vi "9401PWM+with+Midi.vi"() -> ()   [LabVIEW 2013]
uses:
  <vilib>/NIOSC/Argument to Float32 Data.vi
  <vilib>/NIOSC/Generate Error.vi
  <vilib>/FPGAPlugInAG/cRIO-9068/niLvFpga_Open_cRIO-9068.vi
  <vilib>/Utility/error.llb/Error Cluster From Error Code.vi
  <vilib>/rvi/errors/niLvFpgaAdjustHostInterfaceError.vi
  <vilib>/FPGAPlugInAG/cRIO-9068/niLvFpga_Close_cRIO-9068.vi
  <vilib>/rvi/interface/nirviOpenFPGA/nirviOpenFPGA.xnode
  FPGA Bitfiles/testscanmode_FPGATarget_FPGA-PWMExample_nwIUPoe6BIw.lvbitx
  FPGA - PWM Example.vi
  <vilib>/rvi/interface/nirviReadWriteControl/nirviReadWriteControl.xnode
  <vilib>/rvi/interface/nirviCloseFPGA/nirviCloseFPGA.xnode
  <vilib>/NIOSC/NI_OSC.lvlib
  NiFpgaLv.dll
  <vilib>/httpClient/LabVIEWHTTPClient.lvlib
panel:
  in  "Descending (F)":bool
  in  "Priority Columns (0)":i32[](array[numeric])=[1, 2]
  out "error midi parse":errorcluster
  out "duration (min:sec)":string="0:00"
  out "Text":string
  out "Track number: name [channel(s) used]":string="Please select a MIDI file..."
  in  "MIDI file (.mid)":path=path "/home/lvuser/bumble_organ.mid"
  out "error urlfile":errorcluster
  in  "url save file":path=path "/home/lvuser/snoop_dogg-the_shiznit.mid"
  in  "shift":i32(slide)=47 scale=-1.0..107.0
  in  "Array":bool[](array[boolean])
  out "/D59":dbl(slide)=0.5
  out "/D60":dbl(slide)=0.5
  out "/D61":dbl(slide)=0.5
  out "/D62":dbl(slide)=0.5
  out "/D63":dbl(slide)=0.5
  in  "OscBool":bool=TRUE
  in  "MidiBool":bool
  out "/D64":dbl(slide)=0.5
  out "error fpga":errorcluster
  out "/D58":dbl
  out "/D57":dbl
  out "/D56":dbl
  out "/D55":dbl
  out "/D54":dbl
  out "/D53":dbl
  out "/D52":dbl
  out "/D51":dbl
  out "/D50":dbl
  out "/D49":dbl
  out "/D48":dbl
  out "/D47":dbl
  out "/D46":dbl
  out "/D45":dbl
  out "/D44":dbl
  out "/D43":dbl
  out "/D42":dbl
  out "/D41":dbl
  out "/D24":dbl
  out "/D23":dbl
  out "/D22":dbl
  out "/D21":dbl
  out "/D20":dbl
  out "/D19":dbl
  out "/D18":dbl
  out "/D17":dbl
  out "/D16":dbl
  out "/D15":dbl
  out "/D14":dbl
  out "/D13":dbl
  out "/D12":dbl
  out "/D11":dbl
  out "/D10":dbl
  out "/D9":dbl
  out "/D8":dbl
  out "/D7":dbl
  out "/D6":dbl
  out "/D5":dbl
  out "/D4":dbl
  out "/D3":dbl
  out "/D2":dbl
  out "/D40":dbl
  out "/D39":dbl
  out "/D38":dbl
  out "/D37":dbl
  out "/D36":dbl
  out "/D35":dbl
  out "/D34":dbl
  out "/D33":dbl
  out "/D1":dbl
  out "/D32":dbl
  out "/D31":dbl
  out "/D30":dbl
  out "/D29":dbl
  out "/D28":dbl
  out "/D27":dbl
  out "/D25":dbl
  out "/D26":dbl
  out "x .and. y?":bool
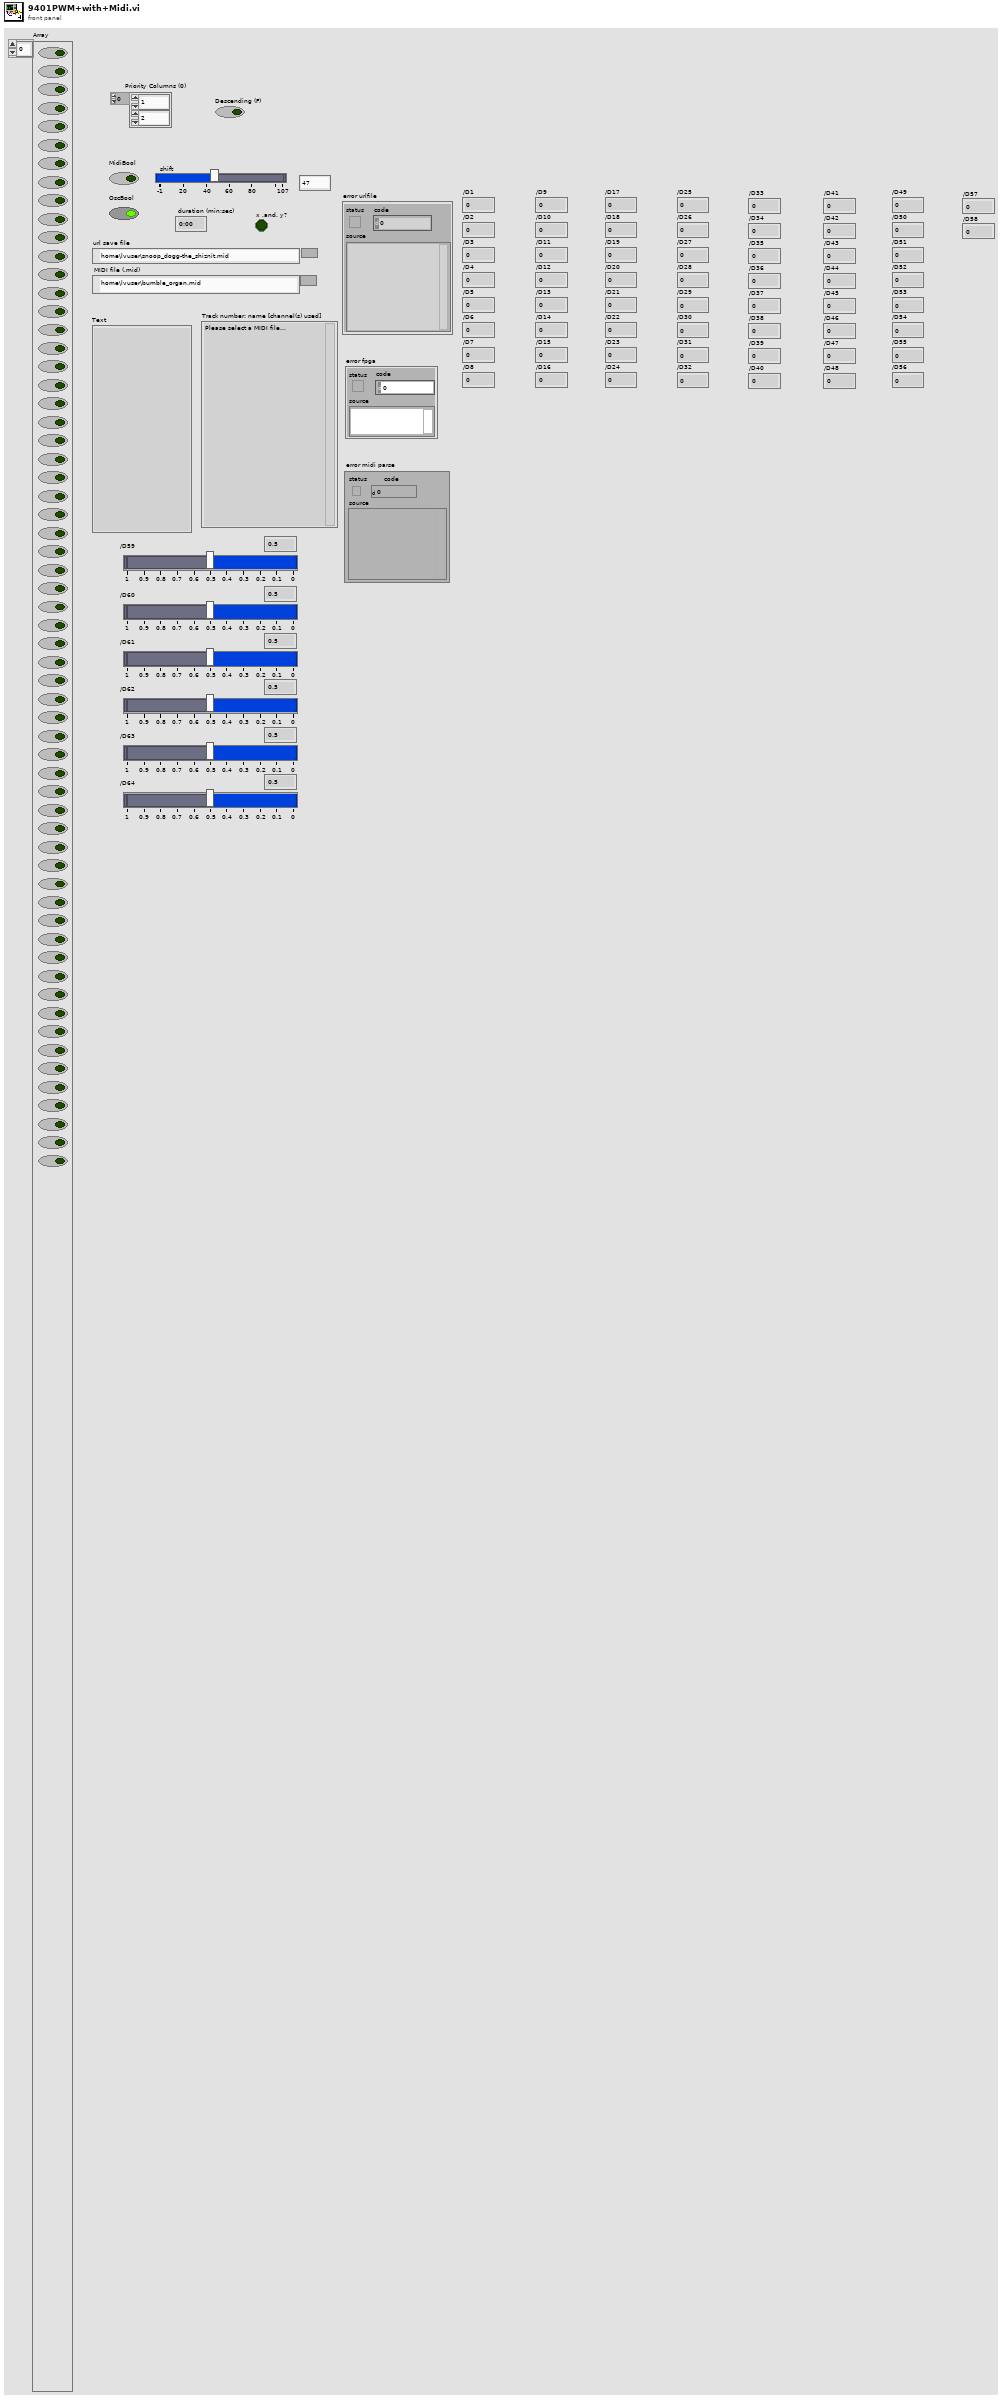
[diagram p1: front panel]
types:
  T1 = typedef "NI_OSC.lvlib/Address Space Node.ctl" = cluster{"parent index":i32, "child indexes":i32[], "address part":string, "method":bool, "data":variant}
  T2 = cluster{"type":u16, "tracks":u16, "ticks per qnote":u16}
  T3 = cluster{"note events":dbl[][], "duration [seconds]":dbl, "track info":string, "text meta-events":string}
  T4 = typedef "NI_OSC.lvlib/Method Dispatching Info.ctl" = cluster{"method address":string, "message":string, "message timetag":u64, "data":variant}
  T5 = typedef "NI_OSC.lvlib/Argument.ctl" = cluster{"argument":string, "type tag":string}
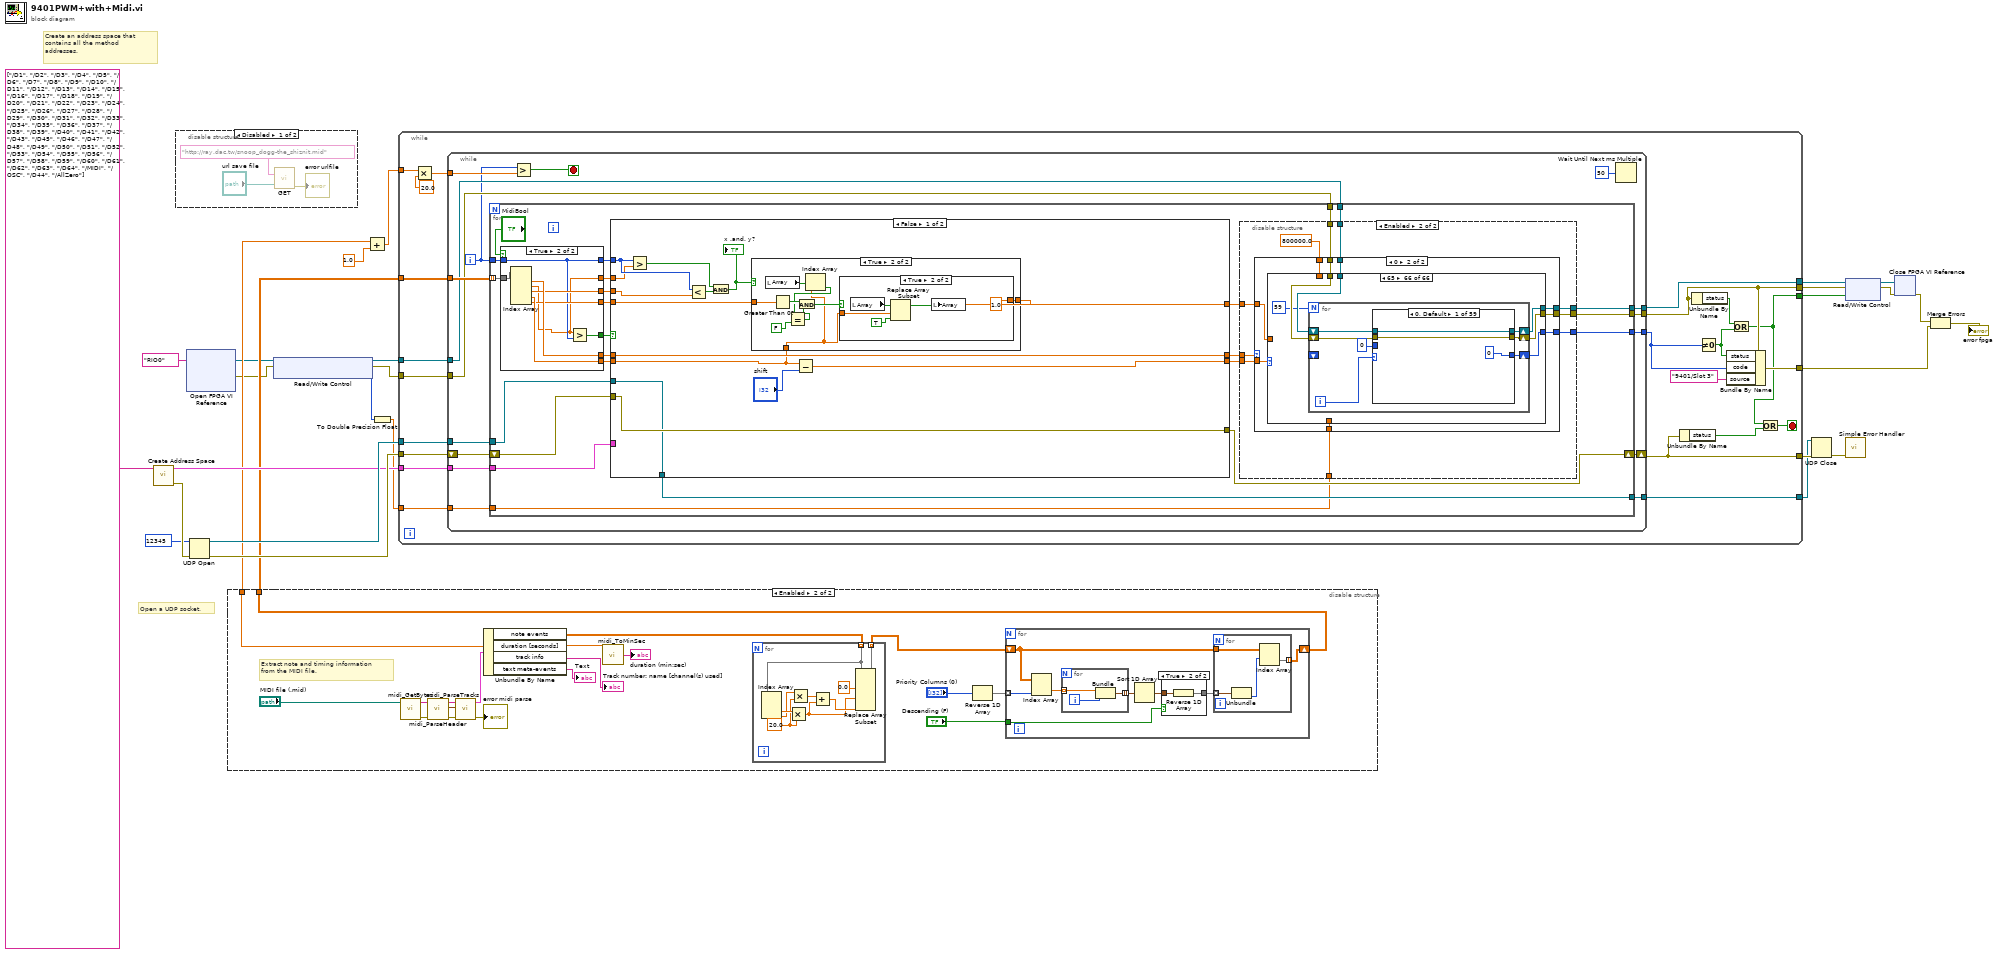
[diagram p0: block diagram]
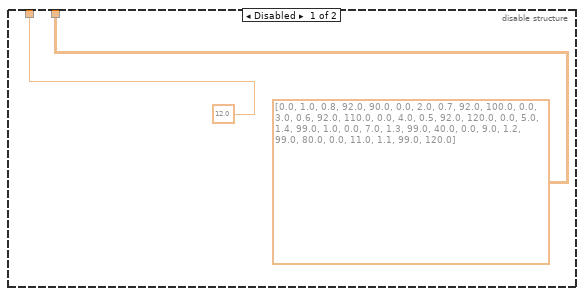
[diagram p3: hidden frame]
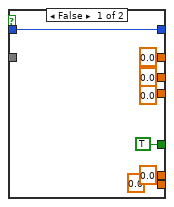
[diagram p5: hidden frame]
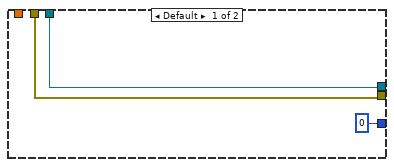
[diagram p7: hidden frame]
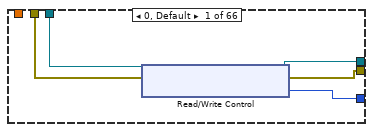
[diagram p8: hidden frame]
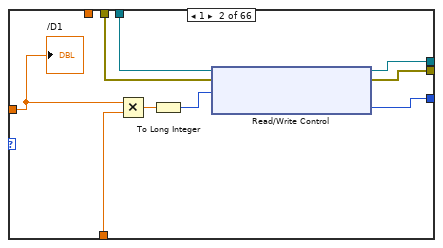
[diagram p9: hidden frame]
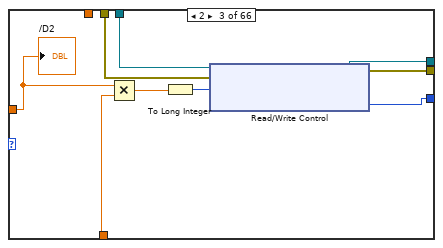
[diagram p10: hidden frame]
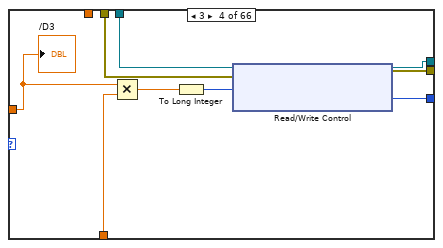
[diagram p11: hidden frame]
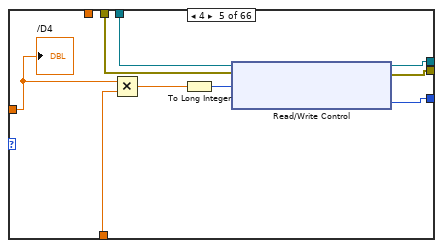
[diagram p12: hidden frame]
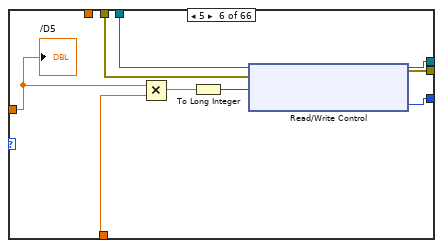
[diagram p13: hidden frame]
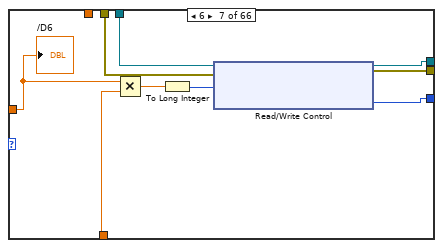
[diagram p14: hidden frame]
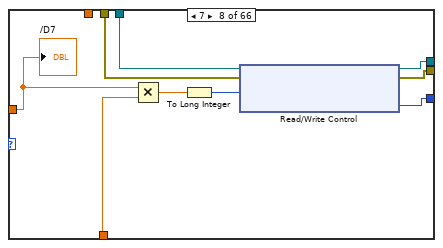
[diagram p15: hidden frame]
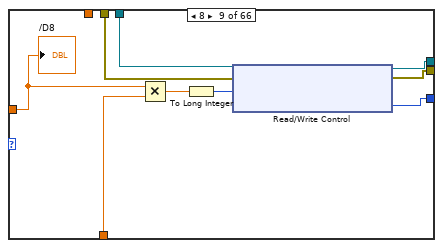
[diagram p16: hidden frame]
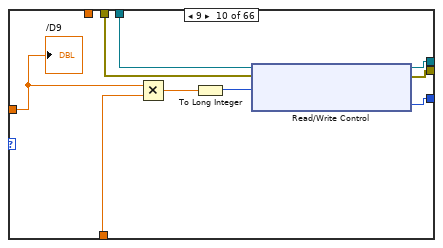
[diagram p17: hidden frame]
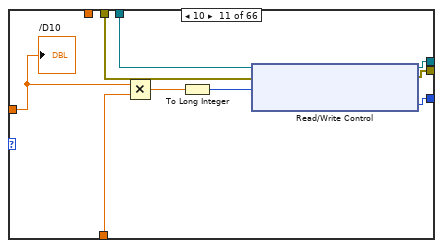
[diagram p18: hidden frame]
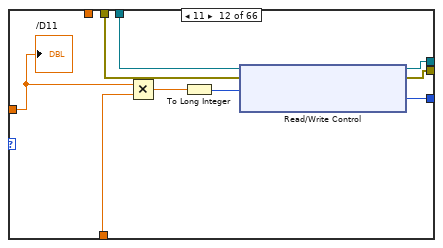
[diagram p19: hidden frame]
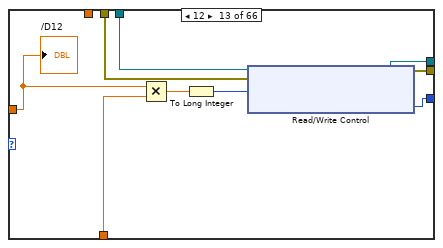
[diagram p20: hidden frame]
diagram:
  # "Open a UDP socket."
  # "Create an address space that contains all the method addresses."
  n1 = call <vilib>:"Create Address Space.vi"("method addresses"=string[] ["/D1", "/D2", "/D3", "/D4", "/D5", "/D6", "/D7", "/D8", "/D9", "/D10", "/D11", "/D12", "/D13", "/D14", "/D15", "/D16", "/D17", "/D18", "/D19", "/D20", "/D21", "/D22", "/D23", "/D24", "/D25", "/D26", "/D27", "/D28", "/D29", "/D30", "/D31", "/D32", "/D33", "/D34", "/D35", "/D36", "/D37", "/D38", "/D39", "/D40", "/D41", "/D42", "/D43", "/D45", "/D46", "/D47", "/D48", "/D49", "/D50", "/D51", "/D52", "/D53", "/D54", "/D55", "/D56", "/D57", "/D58", "/D59", "/D60", "/D61", "/D62", "/D63", "/D64", "/MIDI", "/OSC", "/D44", "/AllZero"]) -> ("error out"=w25:errorcluster, "address space out"=w21:T1[])  [unwired: 9 in]
  n2 = disable-structure shown="Disabled" {
    frame Disabled {
      n3 = call <vilib>:"GET.vi"("output file"="url save file", "url"="http://ray.dac.tw/snoop_dogg-the_shiznit.mid") -> ("error out"=→"error urlfile":errorcluster)  [unwired: 10 in, 3 out]
    }
    frame Enabled {
    }
  }
  n4 = xnode "Open FPGA VI Reference"("resource name"=tag "RIO0") -> ("FPGA VI Reference Out"=w4:refnum<k20>, "error out"=w3:errorcluster)  [unwired: 1 in]
  n5 = UDP Open(8:w25, 11:u16 12345 ("port")) -> (port=w23:refnum<k16>, 0:w22:errorcluster)  [unwired: 3 in, 1 out]
  n6 = disable-structure shown="Enabled" {
    disable-tunnel: [12.0 ("duration [seconds]") w39] -> w20
    disable-tunnel: [dbl[][] [[0.0, 1.0, 0.8, 92.0, 90.0], [0.0, 2.0, 0.7, 92.0, 100.0], [0.0, 3.0, 0.6, 92.0, 110.0], [0.0, 4.0, 0.5, 92.0, 120.0], [0.0, 5.0, 1.4, 99.0, 1.0], [0.0, 7.0, 1.3, 99.0, 40.0], [0.0, 9.0, 1.2, 99.0, 80.0], [0.0, 11.0, 1.1, 99.0, 120.0]] ("note events") w34] -> w19
    frame Disabled {
    }
    frame Enabled {
      # "Extract note and timing information\nfrom the MIDI file."
      n7 = call "midi_GetBytes.vi"("folder name"="MIDI file (.mid)") -> ("error out"=w42:errorcluster, "string"=w49:string)  [unwired: 8 in, 1 out]
      n8 = call "midi_ParseHeader.vi"("error in (no error)"=w42, "string in"=w49) -> ("error out"=w47:errorcluster, "header info"=w43:T2, "string out"=w48:string)  [unwired: 7 in]
      n9 = call "midi_ParseTracks.vi"("error in (no error)"=w47, "header info"=w43, "string in"=w48) -> ("error out"=→"error midi parse":errorcluster, "file contents"=w46:T3)  [unwired: 7 in]
      n10 = Unbundle By Name(w46) -> ("note events"=w40:dbl[][], "duration [seconds]"=w39:dbl, "track info"=→"Track number: name [channel(s) used]":string, "text meta-events"=→"Text":string)
      n11 = call "midi_ToMinSec.vi"("seconds"=w39) -> ("min:sec"=→"duration (min:sec)":string)
      n12 = for {
        tunnel: w40 -> [w76] mode=indexing
        tunnel: [w78] -> w35 mode=indexing
        w74 = 20.0 ("y")
        n13 = Index Array(array=w76) -> (element #2=w75:dbl, element #3=w73:dbl)  [unwired: 3 in, 1 out]
        n14 = Multiply(x=w75, y=w74) -> (x*y=w70:dbl)
        n15 = Multiply(x=w73, y=w74) -> (x*y=w72:dbl)
        n16 = Add(x=w72, y=w70) -> (x+y=w71:dbl)
        n17 = Replace Array Subset(array=w76, new element #1=0.0 ("new element/subarray"), new element #2=w70, new element #3=w71) -> (w78:dbl[])  [unwired: 3 in]
      }
      n18 = Reverse 1D Array(array="Priority Columns (0)") -> (reversed array=w37:i32[])
      n19 = for {
        shift-right: [w53] -> w34
        shift-left: w35 -> [w55]
        tunnel: w37 -> [w52] mode=indexing
        tunnel: "Descending (F)" -> [w54]
        n20 = Index Array(array=w55, index (col)=w52) -> (element=w57:dbl[])  [unwired: 1 in]
        n21 = for {
          tunnel: w57 -> [w67] mode=indexing
          tunnel: [w69] -> w56 mode=indexing
          i -> [w68]
          n22 = Bundle("Numeric"=w67, w68) -> (w69:cluster{"Numeric":dbl, i32})  [unwired: 1 out]
        }
        n23 = Sort 1D Array(array=w56) -> (sorted array=w59:cluster{"Numeric":dbl, i32}[])
        n24 = case shown="True" w54 {
          tunnel: [w60 w61] -> w58
          tunnel: w59 -> [w60 w62]
          frame False {
          }
          frame True {
            n25 = Reverse 1D Array(array=w62) -> (reversed array=w61:cluster{"Numeric":dbl, i32}[])
          }
        }
        n26 = for {
          tunnel: w58 -> [w66] mode=indexing
          tunnel: w55 -> [w65]
          tunnel: [w63] -> w53 mode=indexing
          n27 = Unbundle(w66) -> (w64:i32)  [unwired: 1 out]
          n28 = Index Array(array=w65, index (row)=w64) -> (element=w63:dbl[])  [unwired: 1 in]
        }
      }
    }
  }
  n29 = xnode "Read/Write Control"("FPGA VI Reference In"=w4, "error in"=w3) -> ("FPGA VI Reference Out"=w6:refnum<k20>, "error out"=w5:errorcluster, "PWM Period (Ticks) 0..1"=w2:u32)
  n30 = Add(x=w20, y=1.0) -> (x+y=w28:dbl)
  n31 = To Double Precision Float(number=w2) -> (double precision float=w1:dbl)
  n32 = while {
    tunnel: w19 -> [w100]
    tunnel: w28 -> [w97]
    tunnel: w23 -> [w96]
    tunnel: w22 -> [w95]
    tunnel: w21 -> [w94]
    tunnel: [w80] -> w18
    tunnel: [w93] -> w16
    tunnel: [w89] -> w11
    tunnel: [w88] -> w10
    tunnel: [w82] -> w9
    tunnel: [w86] -> w8
    tunnel: w6 -> [w85]
    tunnel: w5 -> [w84]
    tunnel: w1 -> [w79]
    stop <- w83 stop-if-true
    n33 = Multiply(x=w97, y=20.0) -> (x*y=w98:dbl)
    n34 = while {
      tunnel: w100 -> [w116]
      tunnel: w98 -> [w113]
      tunnel: w94 -> [w110]
      tunnel: w96 -> [w112]
      shift-right: [w109] -> w80
      shift-left: w95 -> [w111]
      tunnel: [w108] -> w93
      tunnel: [w107] -> w88
      tunnel: [w106] -> w89
      tunnel: [w105] -> w87
      tunnel: w85 -> [w104]
      tunnel: w84 -> [w103]
      tunnel: w79 -> [w102]
      i -> [w101]
      stop <- w114 stop-if-true
      n35 = for {
        tunnel: w116 -> [w123] mode=indexing
        tunnel: w101 -> [w125]
        tunnel: w110 -> [w135]
        tunnel: w112 -> [w137]
        shift-right: [w134] -> w109
        shift-left: w111 -> [w136]
        tunnel: [w133] -> w108
        tunnel: [w132] -> w107
        tunnel: [w131] -> w106
        tunnel: [w130] -> w105
        tunnel: w104 -> [w129]
        tunnel: w103 -> [w128]
        tunnel: w102 -> [w127]
        n36 = case shown="True" "MidiBool" {
          tunnel: w125 -> [w147 w149]
          tunnel: [w147 w149] -> w124
          tunnel: w123 -> [_ w155]
          tunnel: [0.0 ("Numeric") w154] -> w122
          tunnel: [0.0 ("Numeric") w153] -> w121
          tunnel: [0.0 w148] -> w120
          tunnel: [0.0 ("Numeric") w152] -> w119
          tunnel: [0.0 ("Numeric") w151] -> w118
          tunnel: [TRUE w150] -> w117
          frame False {
          }
          frame True {
            n37 = Index Array(array=w155) -> (element #1=w153:dbl, element #2=w148:dbl, element #3=w152:dbl, element #4=w154:dbl, element #5=w151:dbl)  [unwired: 5 in]
            n38 = Greater?(x=w148, y=w149) -> (0:w150:bool)
          }
        }
        n39 = case shown="False" w117 {
          tunnel: w118 -> [w1221 _]
          tunnel: w124 -> [w1226 _]
          tunnel: w120 -> [w1225 _]
          tunnel: w119 -> [w1216 _]
          tunnel: w122 -> [w1215 _]
          tunnel: w121 -> [w1218 _]
          tunnel: [w1218 0.0 ("Numeric")] -> w140
          tunnel: [w1217 w1263] -> w139
          tunnel: [w1219 w1259] -> w138
          tunnel: w137 -> [w1223 w1265]
          tunnel: w136 -> [w1224 w1264]
          tunnel: w135 -> [_ w1258]
          tunnel: [w1224 w1262] -> w134
          tunnel: [w1223 w1261] -> w133
          frame False {
            n40 = Greater?(x=w1226, y=w1225) -> (0:w1228:bool)
            n41 = Less?(x=w1226, y=w1216) -> (x < y?=w1227:bool)
            n42 = And(x=w1228, y=w1227) -> (x .and. y?=w1220:bool)
            "x .and. y?" <- w1220
            n43 = case shown="True" w1220 {
              tunnel: w1221 -> [_ w1244]
              tunnel: [w1232 w1241] -> w1219
              tunnel: w1215 -> [w1229 w1240]
              frame False {
                n44 = Index Array(array="Array", index=w1229) -> (element=w1234:bool)
                n45 = Equal?(x=w1234, y=TRUE) -> (x = y?=w1231:bool)
                n46 = case shown="True" w1231 {
                  tunnel: [_ 0.0] -> w1232
                  tunnel: w1229 -> [_ w1238]
                  tunnel: "Array" -> [_ w1237]
                  frame False {
                  }
                  frame True {
                    n47 = Replace Array Subset(array=w1237, new element=FALSE ("new element/subarray"), index=w1238) -> (w1235:bool[])
                    n48 = local write "Array"(w1235) -> ()
                  }
                }
              }
              frame True {
                n49 = local read "Array"() -> (w1248:bool[])
                n50 = Greater Than 0?(x=w1244) -> (x > 0?=w1246:bool)
                n51 = Index Array(array=w1248, index=w1240) -> (element=w1243:bool)
                n52 = Equal?(x=w1243, y=FALSE ("x")) -> (x = y?=w1245:bool)
                n53 = And(x=w1246, y=w1245) -> (x .and. y?=w1247:bool)
                n54 = case shown="True" w1247 {
                  tunnel: [_ 1.0] -> w1241
                  tunnel: w1240 -> [_ w1249]
                  frame False {
                  }
                  frame True {
                    n55 = local read "Array"() -> (w1251:bool[])
                    n56 = Replace Array Subset(array=w1251, new element=TRUE ("new element/subarray"), index=w1249) -> (w1250:bool[])
                    n57 = local write "Array"(w1250) -> ()
                  }
                }
              }
            }
            n58 = Subtract(x=w1215, y="shift") -> (x-y=w1217:dbl)
          }
          frame True {
            n59 = UDP Read(connection ID=w1265, timeout ms (25000)=0, 8:w1264) -> (data out=w1257:string, error out=w1256:errorcluster, 3:w1261:refnum<k16>)  [unwired: 1 in, 2 out]
            n60 = call <vilib>:"Dispatch All Messages.vi"("error in"=w1256, "packet"=w1257, "address space in"=w1258) -> ("error out"=w1255:errorcluster, "method dispatching info"=w1254:T4[])  [unwired: 6 in, 1 out]
            n61 = case shown="No Error" w1255 {
              selector: w1255 -> [w1268 w2007]
              tunnel: [w1272 w2006] -> w1262
              tunnel: [w1271 0] -> w1260
              tunnel: [w1270 0] -> w1263
              tunnel: w1254 -> [w1269 _]
              frame No Error {
                # "Find all method addresses that match the incoming message(s)."
                n62 = for {
                  tunnel: w1269 -> [w1279] mode=indexing
                  shift-right: [w1277] -> w1272
                  shift-left: w1268 -> [w1278]
                  tunnel: [w1274] -> w1271
                  tunnel: [w1273] -> w1270
                  n63 = Unbundle By Name(w1279) -> ("method address"=w1276:string, "message"=w1275:string)
                  n64 = case shown="\"/AllZero\"" w1276 {
                    tunnel: w1278 -> [w1282 w1291 w1302 w1313 w1324 w1335 w1346 w1357 w1368 w1374 w1385 w1397 w1409 w1419 w1430 w1440 w1452 w1464 w1474 w1485 w1496 w1507 w1518 w1529 w1540 w1551 w1562 w1573 w1584 w1595 w1606 w1617 w1628 w1639 w1650 w1661 w1672 w1683 w1694 w1705 w1716 w1727 w1738 w1749 w1760 w1771 w1782 w1793 w1804 w1815 w1825 w1836 w1848 w1858 w1869 w1881 w1891 w1902 w1913 w1923 w1931 w1939 w1947 w1955 w1964 w1974 w1986 w1998]
                    tunnel: [w1282 w1287 w1298 w1309 w1320 w1331 w1342 w1353 w1363 w1376 w1387 w1396 w1408 w1418 w1429 w1442 w1451 w1462 w1473 w1484 w1495 w1506 w1517 w1528 w1539 w1550 w1561 w1572 w1583 w1594 w1605 w1616 w1627 w1638 w1649 w1660 w1671 w1682 w1693 w1704 w1715 w1726 w1737 w1748 w1759 w1770 w1781 w1792 w1803 w1814 w1827 w1838 w1849 w1860 w1871 w1882 w1893 w1904 w1915 w1925 w1933 w1941 w1949 w1957 w1965 w1973 w1985 w1997] -> w1277
                    tunnel: w1275 -> [_ w1286 w1297 w1308 w1319 w1330 w1341 w1352 w1365 w1375 w1386 w1398 w1407 w1420 w1431 w1441 w1453 w1463 w1475 w1486 w1497 w1508 w1519 w1530 w1541 w1552 w1563 w1574 w1585 w1596 w1607 w1618 w1629 w1640 w1651 w1662 w1673 w1684 w1695 w1706 w1717 w1728 w1739 w1750 w1761 w1772 w1783 w1794 w1805 w1816 w1826 w1837 w1847 w1859 w1870 w1880 w1892 w1903 w1914 w1924 w1932 w1940 w1948 w1956 w1963 w1975 w1987 w1996]
                    tunnel: [0 ("int32 data") w1283 w1294 w1305 w1316 w1327 w1338 w1349 w1360 w1371 w1382 w1393 w1404 w1415 w1426 w1437 w1448 w1459 w1470 w1481 w1492 w1503 w1514 w1525 w1536 w1547 w1558 w1569 w1580 w1591 w1602 w1613 w1624 w1635 w1646 w1657 w1668 w1679 w1690 w1701 w1712 w1723 w1734 w1745 w1756 w1767 w1778 w1789 w1800 w1811 w1822 w1833 w1844 w1855 w1866 w1877 w1888 w1899 w1910 w1921 w1929 w1938 w1946 w1954 w1961 0 ("int32 data") 0 ("int32 data") w1994] -> w1274
                    tunnel: [0 w1285 w1296 w1307 w1318 w1328 w1340 w1351 w1362 w1373 w1384 w1395 w1406 w1417 w1428 w1439 w1449 w1461 w1472 w1483 w1494 w1505 w1516 w1527 w1538 w1549 w1560 w1571 w1582 w1593 w1604 w1615 w1626 w1637 w1648 w1659 w1670 w1681 w1692 w1703 w1714 w1725 w1736 w1747 w1758 w1769 w1780 w1791 w1802 w1813 w1824 w1835 w1846 w1857 w1868 w1878 w1889 w1900 w1911 59 60 61 62 63 64 0 0 w1995] -> w1273
                    frame Default {
                    }
                    frame "/D1" {
                      n65 = call <vilib>:"Parse Message.vi"("error in"=w1291, "message"=w1286) -> ("error out"=w1288:errorcluster, "arguments"=w1290:T5[])  [unwired: 7 in, 1 out]
                      n66 = Index Array(array=w1290) -> (element=w1289:T5)  [unwired: 1 in]
                      n67 = call-poly <vilib>:"Argument to Data.vi"("error in"=w1288, "float32 argument"=w1289) -> ("error out"=w1287:errorcluster, "float32 data"=w1283:sgl)  [unwired: 8 in]
                      n68 = local read "OscBool"() -> (w1284:bool)
                      n69 = case shown="True" w1284 {
                        tunnel: [0 1] -> w1285
                        frame False {
                        }
                        frame True {
                        }
                      }
                    }
                    frame "/D2" {
                      n70 = call <vilib>:"Parse Message.vi"("error in"=w1302, "message"=w1297) -> ("error out"=w1299:errorcluster, "arguments"=w1301:T5[])  [unwired: 7 in, 1 out]
                      n71 = Index Array(array=w1301) -> (element=w1300:T5)  [unwired: 1 in]
                      n72 = call-poly <vilib>:"Argument to Data.vi"("error in"=w1299, "float32 argument"=w1300) -> ("error out"=w1298:errorcluster, "float32 data"=w1294:sgl)  [unwired: 8 in]
                      n73 = local read "OscBool"() -> (w1295:bool)
                      n74 = case shown="True" w1295 {
                        tunnel: [0 2] -> w1296
                        frame False {
                        }
                        frame True {
                        }
                      }
                    }
                    frame "/D3" {
                      n75 = local read "OscBool"() -> (w1306:bool)
                      n76 = call <vilib>:"Parse Message.vi"("error in"=w1313, "message"=w1308) -> ("error out"=w1310:errorcluster, "arguments"=w1312:T5[])  [unwired: 7 in, 1 out]
                      n77 = Index Array(array=w1312) -> (element=w1311:T5)  [unwired: 1 in]
                      n78 = case shown="False" w1306 {
                        tunnel: [0 3] -> w1307
                        frame False {
                        }
                        frame True {
                        }
                      }
                      n79 = call-poly <vilib>:"Argument to Data.vi"("error in"=w1310, "float32 argument"=w1311) -> ("error out"=w1309:errorcluster, "float32 data"=w1305:sgl)  [unwired: 8 in]
                    }
                    frame "/D4" {
                      n80 = local read "OscBool"() -> (w1317:bool)
                      n81 = call <vilib>:"Parse Message.vi"("error in"=w1324, "message"=w1319) -> ("error out"=w1321:errorcluster, "arguments"=w1323:T5[])  [unwired: 7 in, 1 out]
                      n82 = Index Array(array=w1323) -> (element=w1322:T5)  [unwired: 1 in]
                      n83 = case shown="True" w1317 {
                        tunnel: [0 4] -> w1318
                        frame False {
                        }
                        frame True {
                        }
                      }
                      n84 = call-poly <vilib>:"Argument to Data.vi"("error in"=w1321, "float32 argument"=w1322) -> ("error out"=w1320:errorcluster, "float32 data"=w1316:sgl)  [unwired: 8 in]
                    }
                    frame "/D5" {
                      n85 = call <vilib>:"Parse Message.vi"("error in"=w1335, "message"=w1330) -> ("error out"=w1332:errorcluster, "arguments"=w1334:T5[])  [unwired: 7 in, 1 out]
                      n86 = Index Array(array=w1334) -> (element=w1333:T5)  [unwired: 1 in]
                      n87 = call-poly <vilib>:"Argument to Data.vi"("error in"=w1332, "float32 argument"=w1333) -> ("error out"=w1331:errorcluster, "float32 data"=w1327:sgl)  [unwired: 8 in]
                      n88 = local read "OscBool"() -> (w1329:bool)
                      n89 = case shown="True" w1329 {
                        tunnel: [0 5] -> w1328
                        frame False {
                        }
                        frame True {
                        }
                      }
                    }
                    frame "/D6" {
                      n90 = call <vilib>:"Parse Message.vi"("error in"=w1346, "message"=w1341) -> ("error out"=w1343:errorcluster, "arguments"=w1345:T5[])  [unwired: 7 in, 1 out]
                      n91 = Index Array(array=w1345) -> (element=w1344:T5)  [unwired: 1 in]
                      n92 = call-poly <vilib>:"Argument to Data.vi"("error in"=w1343, "float32 argument"=w1344) -> ("error out"=w1342:errorcluster, "float32 data"=w1338:sgl)  [unwired: 8 in]
                      n93 = local read "OscBool"() -> (w1339:bool)
                      n94 = case shown="True" w1339 {
                        tunnel: [0 6] -> w1340
                        frame False {
                        }
                        frame True {
                        }
                      }
                    }
                    frame "/D7" {
                      n95 = local read "OscBool"() -> (w1350:bool)
                      n96 = call <vilib>:"Parse Message.vi"("error in"=w1357, "message"=w1352) -> ("error out"=w1354:errorcluster, "arguments"=w1356:T5[])  [unwired: 7 in, 1 out]
                      n97 = Index Array(array=w1356) -> (element=w1355:T5)  [unwired: 1 in]
                      n98 = case shown="True" w1350 {
                        tunnel: [0 7] -> w1351
                        frame False {
                        }
                        frame True {
                        }
                      }
                      n99 = call-poly <vilib>:"Argument to Data.vi"("error in"=w1354, "float32 argument"=w1355) -> ("error out"=w1353:errorcluster, "float32 data"=w1349:sgl)  [unwired: 8 in]
                    }
                    frame "/D8" {
                      n100 = call <vilib>:"Parse Message.vi"("error in"=w1368, "message"=w1365) -> ("error out"=w1364:errorcluster, "arguments"=w1367:T5[])  [unwired: 7 in, 1 out]
                      n101 = local read "OscBool"() -> (w1361:bool)
                      n102 = Index Array(array=w1367) -> (element=w1366:T5)  [unwired: 1 in]
                      n103 = case shown="True" w1361 {
                        tunnel: [0 8] -> w1362
                        frame False {
                        }
                        frame True {
                        }
                      }
                      n104 = call-poly <vilib>:"Argument to Data.vi"("error in"=w1364, "float32 argument"=w1366) -> ("error out"=w1363:errorcluster, "float32 data"=w1360:sgl)  [unwired: 8 in]
                    }
                    frame "/D9" {
                      n105 = local read "OscBool"() -> (w1372:bool)
                      n106 = call <vilib>:"Parse Message.vi"("error in"=w1374, "message"=w1375) -> ("error out"=w1377:errorcluster, "arguments"=w1379:T5[])  [unwired: 7 in, 1 out]
                      n107 = case shown="True" w1372 {
                        tunnel: [0 9] -> w1373
                        frame False {
                        }
                        frame True {
                        }
                      }
                      n108 = Index Array(array=w1379) -> (element=w1378:T5)  [unwired: 1 in]
                      n109 = call-poly <vilib>:"Argument to Data.vi"("error in"=w1377, "float32 argument"=w1378) -> ("error out"=w1376:errorcluster, "float32 data"=w1371:sgl)  [unwired: 8 in]
                    }
                    frame "/D10" {
                      n110 = local read "OscBool"() -> (w1383:bool)
                      n111 = call <vilib>:"Parse Message.vi"("error in"=w1385, "message"=w1386) -> ("error out"=w1390:errorcluster, "arguments"=w1388:T5[])  [unwired: 7 in, 1 out]
                      n112 = case shown="True" w1383 {
                        tunnel: [0 10] -> w1384
                        frame False {
                        }
                        frame True {
                        }
                      }
                      n113 = Index Array(array=w1388) -> (element=w1389:T5)  [unwired: 1 in]
                      n114 = call-poly <vilib>:"Argument to Data.vi"("error in"=w1390, "float32 argument"=w1389) -> ("error out"=w1387:errorcluster, "float32 data"=w1382:sgl)  [unwired: 8 in]
                    }
                    frame "/D11" {
                      n115 = local read "OscBool"() -> (w1394:bool)
                      n116 = call <vilib>:"Parse Message.vi"("error in"=w1397, "message"=w1398) -> ("error out"=w1399:errorcluster, "arguments"=w1401:T5[])  [unwired: 7 in, 1 out]
                      n117 = case shown="True" w1394 {
                        tunnel: [0 11] -> w1395
                        frame False {
                        }
                        frame True {
                        }
                      }
                      n118 = Index Array(array=w1401) -> (element=w1400:T5)  [unwired: 1 in]
                      n119 = call-poly <vilib>:"Argument to Data.vi"("error in"=w1399, "float32 argument"=w1400) -> ("error out"=w1396:errorcluster, "float32 data"=w1393:sgl)  [unwired: 8 in]
                    }
                    frame "/D12" {
                      n120 = local read "OscBool"() -> (w1405:bool)
                      n121 = call <vilib>:"Parse Message.vi"("error in"=w1409, "message"=w1407) -> ("error out"=w1410:errorcluster, "arguments"=w1412:T5[])  [unwired: 7 in, 1 out]
                      n122 = case shown="True" w1405 {
                        tunnel: [0 12] -> w1406
                        frame False {
                        }
                        frame True {
                        }
                      }
                      n123 = Index Array(array=w1412) -> (element=w1411:T5)  [unwired: 1 in]
                      n124 = call-poly <vilib>:"Argument to Data.vi"("error in"=w1410, "float32 argument"=w1411) -> ("error out"=w1408:errorcluster, "float32 data"=w1404:sgl)  [unwired: 8 in]
                    }
                    frame "/D13" {
                      n125 = local read "OscBool"() -> (w1416:bool)
                      n126 = call <vilib>:"Parse Message.vi"("error in"=w1419, "message"=w1420) -> ("error out"=w1423:errorcluster, "arguments"=w1421:T5[])  [unwired: 7 in, 1 out]
                      n127 = case shown="True" w1416 {
                        tunnel: [0 13] -> w1417
                        frame False {
                        }
                        frame True {
                        }
                      }
                      n128 = Index Array(array=w1421) -> (element=w1422:T5)  [unwired: 1 in]
                      n129 = call-poly <vilib>:"Argument to Data.vi"("error in"=w1423, "float32 argument"=w1422) -> ("error out"=w1418:errorcluster, "float32 data"=w1415:sgl)  [unwired: 8 in]
                    }
                    frame "/D14" {
                      n130 = local read "OscBool"() -> (w1427:bool)
                      n131 = call <vilib>:"Parse Message.vi"("error in"=w1430, "message"=w1431) -> ("error out"=w1434:errorcluster, "arguments"=w1432:T5[])  [unwired: 7 in, 1 out]
                      n132 = case shown="True" w1427 {
                        tunnel: [0 14] -> w1428
                        frame False {
                        }
                        frame True {
                        }
                      }
                      n133 = Index Array(array=w1432) -> (element=w1433:T5)  [unwired: 1 in]
                      n134 = call-poly <vilib>:"Argument to Data.vi"("error in"=w1434, "float32 argument"=w1433) -> ("error out"=w1429:errorcluster, "float32 data"=w1426:sgl)  [unwired: 8 in]
                    }
                    frame "/D15" {
                      n135 = local read "OscBool"() -> (w1438:bool)
                      n136 = call <vilib>:"Parse Message.vi"("error in"=w1440, "message"=w1441) -> ("error out"=w1443:errorcluster, "arguments"=w1445:T5[])  [unwired: 7 in, 1 out]
                      n137 = case shown="True" w1438 {
                        tunnel: [0 15] -> w1439
                        frame False {
                        }
                        frame True {
                        }
                      }
                      n138 = Index Array(array=w1445) -> (element=w1444:T5)  [unwired: 1 in]
                      n139 = call-poly <vilib>:"Argument to Data.vi"("error in"=w1443, "float32 argument"=w1444) -> ("error out"=w1442:errorcluster, "float32 data"=w1437:sgl)  [unwired: 8 in]
                    }
                    frame "/D16" {
                      n140 = local read "OscBool"() -> (w1450:bool)
                      n141 = call <vilib>:"Parse Message.vi"("error in"=w1452, "message"=w1453) -> ("error out"=w1454:errorcluster, "arguments"=w1456:T5[])  [unwired: 7 in, 1 out]
                      n142 = case shown="True" w1450 {
                        tunnel: [0 16] -> w1449
                        frame False {
                        }
                        frame True {
                        }
                      }
                      n143 = Index Array(array=w1456) -> (element=w1455:T5)  [unwired: 1 in]
                      n144 = call-poly <vilib>:"Argument to Data.vi"("error in"=w1454, "float32 argument"=w1455) -> ("error out"=w1451:errorcluster, "float32 data"=w1448:sgl)  [unwired: 8 in]
                    }
                    frame "/D17" {
                      n145 = local read "OscBool"() -> (w1460:bool)
                      n146 = call <vilib>:"Parse Message.vi"("error in"=w1464, "message"=w1463) -> ("error out"=w1465:errorcluster, "arguments"=w1467:T5[])  [unwired: 7 in, 1 out]
                      n147 = case shown="True" w1460 {
                        tunnel: [0 17] -> w1461
                        frame False {
                        }
                        frame True {
                        }
                      }
                      n148 = Index Array(array=w1467) -> (element=w1466:T5)  [unwired: 1 in]
                      n149 = call-poly <vilib>:"Argument to Data.vi"("error in"=w1465, "float32 argument"=w1466) -> ("error out"=w1462:errorcluster, "float32 data"=w1459:sgl)  [unwired: 8 in]
                    }
                    frame "/D18" {
                      n150 = local read "OscBool"() -> (w1471:bool)
                      n151 = call <vilib>:"Parse Message.vi"("error in"=w1474, "message"=w1475) -> ("error out"=w1476:errorcluster, "arguments"=w1478:T5[])  [unwired: 7 in, 1 out]
                      n152 = case shown="True" w1471 {
                        tunnel: [0 18] -> w1472
                        frame False {
                        }
                        frame True {
                        }
                      }
                      n153 = Index Array(array=w1478) -> (element=w1477:T5)  [unwired: 1 in]
                      n154 = call-poly <vilib>:"Argument to Data.vi"("error in"=w1476, "float32 argument"=w1477) -> ("error out"=w1473:errorcluster, "float32 data"=w1470:sgl)  [unwired: 8 in]
                    }
                    frame "/D19" {
                      n155 = local read "OscBool"() -> (w1482:bool)
                      n156 = call <vilib>:"Parse Message.vi"("error in"=w1485, "message"=w1486) -> ("error out"=w1487:errorcluster, "arguments"=w1489:T5[])  [unwired: 7 in, 1 out]
                      n157 = case shown="True" w1482 {
                        tunnel: [0 19] -> w1483
                        frame False {
                        }
                        frame True {
                        }
                      }
                      n158 = Index Array(array=w1489) -> (element=w1488:T5)  [unwired: 1 in]
                      n159 = call-poly <vilib>:"Argument to Data.vi"("error in"=w1487, "float32 argument"=w1488) -> ("error out"=w1484:errorcluster, "float32 data"=w1481:sgl)  [unwired: 8 in]
                    }
                    frame "/D20" {
                      n160 = local read "OscBool"() -> (w1493:bool)
                      n161 = call <vilib>:"Parse Message.vi"("error in"=w1496, "message"=w1497) -> ("error out"=w1498:errorcluster, "arguments"=w1500:T5[])  [unwired: 7 in, 1 out]
                      n162 = case shown="False" w1493 {
                        tunnel: [0 20] -> w1494
                        frame False {
                        }
                        frame True {
                        }
                      }
                      n163 = Index Array(array=w1500) -> (element=w1499:T5)  [unwired: 1 in]
                      n164 = call-poly <vilib>:"Argument to Data.vi"("error in"=w1498, "float32 argument"=w1499) -> ("error out"=w1495:errorcluster, "float32 data"=w1492:sgl)  [unwired: 8 in]
                    }
                    frame "/D21" {
                      n165 = local read "OscBool"() -> (w1504:bool)
                      n166 = call <vilib>:"Parse Message.vi"("error in"=w1507, "message"=w1508) -> ("error out"=w1509:errorcluster, "arguments"=w1511:T5[])  [unwired: 7 in, 1 out]
                      n167 = case shown="True" w1504 {
                        tunnel: [0 21] -> w1505
                        frame False {
                        }
                        frame True {
                        }
                      }
                      n168 = Index Array(array=w1511) -> (element=w1510:T5)  [unwired: 1 in]
                      n169 = call-poly <vilib>:"Argument to Data.vi"("error in"=w1509, "float32 argument"=w1510) -> ("error out"=w1506:errorcluster, "float32 data"=w1503:sgl)  [unwired: 8 in]
                    }
                    frame "/D22" {
                      n170 = local read "OscBool"() -> (w1515:bool)
                      n171 = call <vilib>:"Parse Message.vi"("error in"=w1518, "message"=w1519) -> ("error out"=w1520:errorcluster, "arguments"=w1522:T5[])  [unwired: 7 in, 1 out]
                      n172 = case shown="True" w1515 {
                        tunnel: [0 22] -> w1516
                        frame False {
                        }
                        frame True {
                        }
                      }
                      n173 = Index Array(array=w1522) -> (element=w1521:T5)  [unwired: 1 in]
                      n174 = call-poly <vilib>:"Argument to Data.vi"("error in"=w1520, "float32 argument"=w1521) -> ("error out"=w1517:errorcluster, "float32 data"=w1514:sgl)  [unwired: 8 in]
                    }
                    frame "/D23" {
                      n175 = local read "OscBool"() -> (w1526:bool)
                      n176 = call <vilib>:"Parse Message.vi"("error in"=w1529, "message"=w1530) -> ("error out"=w1533:errorcluster, "arguments"=w1531:T5[])  [unwired: 7 in, 1 out]
                      n177 = case shown="True" w1526 {
                        tunnel: [0 23] -> w1527
                        frame False {
                        }
                        frame True {
                        }
                      }
                      n178 = Index Array(array=w1531) -> (element=w1532:T5)  [unwired: 1 in]
                      n179 = call-poly <vilib>:"Argument to Data.vi"("error in"=w1533, "float32 argument"=w1532) -> ("error out"=w1528:errorcluster, "float32 data"=w1525:sgl)  [unwired: 8 in]
                    }
                    frame "/D24" {
                      n180 = local read "OscBool"() -> (w1537:bool)
                      n181 = call <vilib>:"Parse Message.vi"("error in"=w1540, "message"=w1541) -> ("error out"=w1542:errorcluster, "arguments"=w1544:T5[])  [unwired: 7 in, 1 out]
                      n182 = case shown="True" w1537 {
                        tunnel: [0 24] -> w1538
                        frame False {
                        }
                        frame True {
                        }
                      }
                      n183 = Index Array(array=w1544) -> (element=w1543:T5)  [unwired: 1 in]
                      n184 = call-poly <vilib>:"Argument to Data.vi"("error in"=w1542, "float32 argument"=w1543) -> ("error out"=w1539:errorcluster, "float32 data"=w1536:sgl)  [unwired: 8 in]
                    }
                    frame "/D25" {
                      n185 = local read "OscBool"() -> (w1548:bool)
                      n186 = call <vilib>:"Parse Message.vi"("error in"=w1551, "message"=w1552) -> ("error out"=w1555:errorcluster, "arguments"=w1553:T5[])  [unwired: 7 in, 1 out]
                      n187 = case shown="True" w1548 {
                        tunnel: [0 25] -> w1549
                        frame False {
                        }
                        frame True {
                        }
                      }
                      n188 = Index Array(array=w1553) -> (element=w1554:T5)  [unwired: 1 in]
                      n189 = call-poly <vilib>:"Argument to Data.vi"("error in"=w1555, "float32 argument"=w1554) -> ("error out"=w1550:errorcluster, "float32 data"=w1547:sgl)  [unwired: 8 in]
                    }
                    frame "/D26" {
                      n190 = local read "OscBool"() -> (w1559:bool)
                      n191 = call <vilib>:"Parse Message.vi"("error in"=w1562, "message"=w1563) -> ("error out"=w1564:errorcluster, "arguments"=w1566:T5[])  [unwired: 7 in, 1 out]
                      n192 = case shown="True" w1559 {
                        tunnel: [0 26] -> w1560
                        frame False {
                        }
                        frame True {
                        }
                      }
                      n193 = Index Array(array=w1566) -> (element=w1565:T5)  [unwired: 1 in]
                      n194 = call-poly <vilib>:"Argument to Data.vi"("error in"=w1564, "float32 argument"=w1565) -> ("error out"=w1561:errorcluster, "float32 data"=w1558:sgl)  [unwired: 8 in]
                    }
                    frame "/D27" {
                      n195 = local read "OscBool"() -> (w1570:bool)
                      n196 = call <vilib>:"Parse Message.vi"("error in"=w1573, "message"=w1574) -> ("error out"=w1577:errorcluster, "arguments"=w1575:T5[])  [unwired: 7 in, 1 out]
                      n197 = case shown="True" w1570 {
                        tunnel: [0 27] -> w1571
                        frame False {
                        }
                        frame True {
                        }
                      }
                      n198 = Index Array(array=w1575) -> (element=w1576:T5)  [unwired: 1 in]
                      n199 = call-poly <vilib>:"Argument to Data.vi"("error in"=w1577, "float32 argument"=w1576) -> ("error out"=w1572:errorcluster, "float32 data"=w1569:sgl)  [unwired: 8 in]
                    }
                    frame "/D28" {
                      n200 = local read "OscBool"() -> (w1581:bool)
                      n201 = call <vilib>:"Parse Message.vi"("error in"=w1584, "message"=w1585) -> ("error out"=w1588:errorcluster, "arguments"=w1586:T5[])  [unwired: 7 in, 1 out]
                      n202 = case shown="True" w1581 {
                        tunnel: [0 28] -> w1582
                        frame False {
                        }
                        frame True {
                        }
                      }
                      n203 = Index Array(array=w1586) -> (element=w1587:T5)  [unwired: 1 in]
                      n204 = call-poly <vilib>:"Argument to Data.vi"("error in"=w1588, "float32 argument"=w1587) -> ("error out"=w1583:errorcluster, "float32 data"=w1580:sgl)  [unwired: 8 in]
                    }
                    frame "/D29" {
                      n205 = local read "OscBool"() -> (w1592:bool)
                      n206 = call <vilib>:"Parse Message.vi"("error in"=w1595, "message"=w1596) -> ("error out"=w1597:errorcluster, "arguments"=w1599:T5[])  [unwired: 7 in, 1 out]
                      n207 = case shown="True" w1592 {
                        tunnel: [0 29] -> w1593
                        frame False {
                        }
                        frame True {
                        }
                      }
                      n208 = Index Array(array=w1599) -> (element=w1598:T5)  [unwired: 1 in]
                      n209 = call-poly <vilib>:"Argument to Data.vi"("error in"=w1597, "float32 argument"=w1598) -> ("error out"=w1594:errorcluster, "float32 data"=w1591:sgl)  [unwired: 8 in]
                    }
                    frame "/D30" {
                      n210 = local read "OscBool"() -> (w1603:bool)
                      n211 = call <vilib>:"Parse Message.vi"("error in"=w1606, "message"=w1607) -> ("error out"=w1608:errorcluster, "arguments"=w1610:T5[])  [unwired: 7 in, 1 out]
                      n212 = case shown="True" w1603 {
                        tunnel: [0 30] -> w1604
                        frame False {
                        }
                        frame True {
                        }
                      }
                      n213 = Index Array(array=w1610) -> (element=w1609:T5)  [unwired: 1 in]
                      n214 = call-poly <vilib>:"Argument to Data.vi"("error in"=w1608, "float32 argument"=w1609) -> ("error out"=w1605:errorcluster, "float32 data"=w1602:sgl)  [unwired: 8 in]
                    }
                    frame "/D31" {
                      n215 = local read "OscBool"() -> (w1614:bool)
                      n216 = call <vilib>:"Parse Message.vi"("error in"=w1617, "message"=w1618) -> ("error out"=w1619:errorcluster, "arguments"=w1621:T5[])  [unwired: 7 in, 1 out]
                      n217 = case shown="True" w1614 {
                        tunnel: [0 31] -> w1615
                        frame False {
                        }
                        frame True {
                        }
                      }
                      n218 = Index Array(array=w1621) -> (element=w1620:T5)  [unwired: 1 in]
                      n219 = call-poly <vilib>:"Argument to Data.vi"("error in"=w1619, "float32 argument"=w1620) -> ("error out"=w1616:errorcluster, "float32 data"=w1613:sgl)  [unwired: 8 in]
                    }
                    frame "/D32" {
                      n220 = local read "OscBool"() -> (w1625:bool)
                      n221 = call <vilib>:"Parse Message.vi"("error in"=w1628, "message"=w1629) -> ("error out"=w1630:errorcluster, "arguments"=w1632:T5[])  [unwired: 7 in, 1 out]
                      n222 = case shown="True" w1625 {
                        tunnel: [0 32] -> w1626
                        frame False {
                        }
                        frame True {
                        }
                      }
                      n223 = Index Array(array=w1632) -> (element=w1631:T5)  [unwired: 1 in]
                      n224 = call-poly <vilib>:"Argument to Data.vi"("error in"=w1630, "float32 argument"=w1631) -> ("error out"=w1627:errorcluster, "float32 data"=w1624:sgl)  [unwired: 8 in]
                    }
                    frame "/D33" {
                      n225 = local read "OscBool"() -> (w1636:bool)
                      n226 = call <vilib>:"Parse Message.vi"("error in"=w1639, "message"=w1640) -> ("error out"=w1643:errorcluster, "arguments"=w1641:T5[])  [unwired: 7 in, 1 out]
                      n227 = case shown="True" w1636 {
                        tunnel: [0 33] -> w1637
                        frame False {
                        }
                        frame True {
                        }
                      }
                      n228 = Index Array(array=w1641) -> (element=w1642:T5)  [unwired: 1 in]
                      n229 = call-poly <vilib>:"Argument to Data.vi"("error in"=w1643, "float32 argument"=w1642) -> ("error out"=w1638:errorcluster, "float32 data"=w1635:sgl)  [unwired: 8 in]
                    }
                    frame "/D34" {
                      n230 = local read "OscBool"() -> (w1647:bool)
                      n231 = call <vilib>:"Parse Message.vi"("error in"=w1650, "message"=w1651) -> ("error out"=w1654:errorcluster, "arguments"=w1652:T5[])  [unwired: 7 in, 1 out]
                      n232 = case shown="True" w1647 {
                        tunnel: [0 34] -> w1648
                        frame False {
                        }
                        frame True {
                        }
                      }
                      n233 = Index Array(array=w1652) -> (element=w1653:T5)  [unwired: 1 in]
                      n234 = call-poly <vilib>:"Argument to Data.vi"("error in"=w1654, "float32 argument"=w1653) -> ("error out"=w1649:errorcluster, "float32 data"=w1646:sgl)  [unwired: 8 in]
                    }
                    frame "/D35" {
                      n235 = local read "OscBool"() -> (w1658:bool)
                      n236 = call <vilib>:"Parse Message.vi"("error in"=w1661, "message"=w1662) -> ("error out"=w1663:errorcluster, "arguments"=w1665:T5[])  [unwired: 7 in, 1 out]
                      n237 = case shown="True" w1658 {
                        tunnel: [0 35] -> w1659
                        frame False {
                        }
                        frame True {
                        }
                      }
                      n238 = Index Array(array=w1665) -> (element=w1664:T5)  [unwired: 1 in]
                      n239 = call-poly <vilib>:"Argument to Data.vi"("error in"=w1663, "float32 argument"=w1664) -> ("error out"=w1660:errorcluster, "float32 data"=w1657:sgl)  [unwired: 8 in]
                    }
                    frame "/D36" {
                      n240 = local read "OscBool"() -> (w1669:bool)
                      n241 = case shown="True" w1669 {
                        tunnel: [0 36] -> w1670
                        frame False {
                        }
                        frame True {
                        }
                      }
                      n242 = call <vilib>:"Parse Message.vi"("error in"=w1672, "message"=w1673) -> ("error out"=w1676:errorcluster, "arguments"=w1674:T5[])  [unwired: 7 in, 1 out]
                      n243 = Index Array(array=w1674) -> (element=w1675:T5)  [unwired: 1 in]
                      n244 = call-poly <vilib>:"Argument to Data.vi"("error in"=w1676, "float32 argument"=w1675) -> ("error out"=w1671:errorcluster, "float32 data"=w1668:sgl)  [unwired: 8 in]
                    }
                    frame "/D37" {
                      n245 = local read "OscBool"() -> (w1680:bool)
                      n246 = case shown="True" w1680 {
                        tunnel: [0 37] -> w1681
                        frame False {
                        }
                        frame True {
                        }
                      }
                      n247 = call <vilib>:"Parse Message.vi"("error in"=w1683, "message"=w1684) -> ("error out"=w1685:errorcluster, "arguments"=w1687:T5[])  [unwired: 7 in, 1 out]
                      n248 = Index Array(array=w1687) -> (element=w1686:T5)  [unwired: 1 in]
                      n249 = call-poly <vilib>:"Argument to Data.vi"("error in"=w1685, "float32 argument"=w1686) -> ("error out"=w1682:errorcluster, "float32 data"=w1679:sgl)  [unwired: 8 in]
                    }
                    frame "/D38" {
                      n250 = local read "OscBool"() -> (w1691:bool)
                      n251 = call <vilib>:"Parse Message.vi"("error in"=w1694, "message"=w1695) -> ("error out"=w1696:errorcluster, "arguments"=w1698:T5[])  [unwired: 7 in, 1 out]
                      n252 = case shown="True" w1691 {
                        tunnel: [0 38] -> w1692
                        frame False {
                        }
                        frame True {
                        }
                      }
                      n253 = Index Array(array=w1698) -> (element=w1697:T5)  [unwired: 1 in]
                      n254 = call-poly <vilib>:"Argument to Data.vi"("error in"=w1696, "float32 argument"=w1697) -> ("error out"=w1693:errorcluster, "float32 data"=w1690:sgl)  [unwired: 8 in]
                    }
                    frame "/D39" {
                      n255 = local read "OscBool"() -> (w1702:bool)
                      n256 = call <vilib>:"Parse Message.vi"("error in"=w1705, "message"=w1706) -> ("error out"=w1707:errorcluster, "arguments"=w1709:T5[])  [unwired: 7 in, 1 out]
                      n257 = case shown="True" w1702 {
                        tunnel: [0 39] -> w1703
                        frame False {
                        }
                        frame True {
                        }
                      }
                      n258 = Index Array(array=w1709) -> (element=w1708:T5)  [unwired: 1 in]
                      n259 = call-poly <vilib>:"Argument to Data.vi"("error in"=w1707, "float32 argument"=w1708) -> ("error out"=w1704:errorcluster, "float32 data"=w1701:sgl)  [unwired: 8 in]
                    }
                    frame "/D40" {
                      n260 = local read "OscBool"() -> (w1713:bool)
                      n261 = call <vilib>:"Parse Message.vi"("error in"=w1716, "message"=w1717) -> ("error out"=w1718:errorcluster, "arguments"=w1720:T5[])  [unwired: 7 in, 1 out]
                      n262 = case shown="True" w1713 {
                        tunnel: [0 40] -> w1714
                        frame False {
                        }
                        frame True {
                        }
                      }
                      n263 = Index Array(array=w1720) -> (element=w1719:T5)  [unwired: 1 in]
                      n264 = call-poly <vilib>:"Argument to Data.vi"("error in"=w1718, "float32 argument"=w1719) -> ("error out"=w1715:errorcluster, "float32 data"=w1712:sgl)  [unwired: 8 in]
                    }
                    frame "/D41" {
                      n265 = local read "OscBool"() -> (w1724:bool)
                      n266 = case shown="True" w1724 {
                        tunnel: [0 41] -> w1725
                        frame False {
                        }
                        frame True {
                        }
                      }
                      n267 = call <vilib>:"Parse Message.vi"("error in"=w1727, "message"=w1728) -> ("error out"=w1729:errorcluster, "arguments"=w1731:T5[])  [unwired: 7 in, 1 out]
                      n268 = Index Array(array=w1731) -> (element=w1730:T5)  [unwired: 1 in]
                      n269 = call-poly <vilib>:"Argument to Data.vi"("error in"=w1729, "float32 argument"=w1730) -> ("error out"=w1726:errorcluster, "float32 data"=w1723:sgl)  [unwired: 8 in]
                    }
                    frame "/D42" {
                      n270 = local read "OscBool"() -> (w1735:bool)
                      n271 = call <vilib>:"Parse Message.vi"("error in"=w1738, "message"=w1739) -> ("error out"=w1742:errorcluster, "arguments"=w1740:T5[])  [unwired: 7 in, 1 out]
                      n272 = case shown="True" w1735 {
                        tunnel: [0 42] -> w1736
                        frame False {
                        }
                        frame True {
                        }
                      }
                      n273 = Index Array(array=w1740) -> (element=w1741:T5)  [unwired: 1 in]
                      n274 = call-poly <vilib>:"Argument to Data.vi"("error in"=w1742, "float32 argument"=w1741) -> ("error out"=w1737:errorcluster, "float32 data"=w1734:sgl)  [unwired: 8 in]
                    }
                    frame "/D43" {
                      n275 = local read "OscBool"() -> (w1746:bool)
                      n276 = call <vilib>:"Parse Message.vi"("error in"=w1749, "message"=w1750) -> ("error out"=w1753:errorcluster, "arguments"=w1751:T5[])  [unwired: 7 in, 1 out]
                      n277 = case shown="True" w1746 {
                        tunnel: [0 43] -> w1747
                        frame False {
                        }
                        frame True {
                        }
                      }
                      n278 = Index Array(array=w1751) -> (element=w1752:T5)  [unwired: 1 in]
                      n279 = call-poly <vilib>:"Argument to Data.vi"("error in"=w1753, "float32 argument"=w1752) -> ("error out"=w1748:errorcluster, "float32 data"=w1745:sgl)  [unwired: 8 in]
                    }
                    frame "/D44" {
                      n280 = local read "OscBool"() -> (w1757:bool)
                      n281 = call <vilib>:"Parse Message.vi"("error in"=w1760, "message"=w1761) -> ("error out"=w1764:errorcluster, "arguments"=w1762:T5[])  [unwired: 7 in, 1 out]
                      n282 = case shown="True" w1757 {
                        tunnel: [0 44] -> w1758
                        frame False {
                        }
                        frame True {
                        }
                      }
                      n283 = Index Array(array=w1762) -> (element=w1763:T5)  [unwired: 1 in]
                      n284 = call-poly <vilib>:"Argument to Data.vi"("error in"=w1764, "float32 argument"=w1763) -> ("error out"=w1759:errorcluster, "float32 data"=w1756:sgl)  [unwired: 8 in]
                    }
                    frame "/D45" {
                      n285 = local read "OscBool"() -> (w1768:bool)
                      n286 = call <vilib>:"Parse Message.vi"("error in"=w1771, "message"=w1772) -> ("error out"=w1773:errorcluster, "arguments"=w1775:T5[])  [unwired: 7 in, 1 out]
                      n287 = case shown="True" w1768 {
                        tunnel: [0 45] -> w1769
                        frame False {
                        }
                        frame True {
                        }
                      }
                      n288 = Index Array(array=w1775) -> (element=w1774:T5)  [unwired: 1 in]
                      n289 = call-poly <vilib>:"Argument to Data.vi"("error in"=w1773, "float32 argument"=w1774) -> ("error out"=w1770:errorcluster, "float32 data"=w1767:sgl)  [unwired: 8 in]
                    }
                    frame "/D46" {
                      n290 = local read "OscBool"() -> (w1779:bool)
                      n291 = call <vilib>:"Parse Message.vi"("error in"=w1782, "message"=w1783) -> ("error out"=w1786:errorcluster, "arguments"=w1784:T5[])  [unwired: 7 in, 1 out]
                      n292 = case shown="True" w1779 {
                        tunnel: [0 46] -> w1780
                        frame False {
                        }
                        frame True {
                        }
                      }
                      n293 = Index Array(array=w1784) -> (element=w1785:T5)  [unwired: 1 in]
                      n294 = call-poly <vilib>:"Argument to Data.vi"("error in"=w1786, "float32 argument"=w1785) -> ("error out"=w1781:errorcluster, "float32 data"=w1778:sgl)  [unwired: 8 in]
                    }
                    frame "/D47" {
                      n295 = local read "OscBool"() -> (w1790:bool)
                      n296 = call <vilib>:"Parse Message.vi"("error in"=w1793, "message"=w1794) -> ("error out"=w1795:errorcluster, "arguments"=w1797:T5[])  [unwired: 7 in, 1 out]
                      n297 = case shown="False" w1790 {
                        tunnel: [0 47] -> w1791
                        frame False {
                        }
                        frame True {
                        }
                      }
                      n298 = Index Array(array=w1797) -> (element=w1796:T5)  [unwired: 1 in]
                      n299 = call-poly <vilib>:"Argument to Data.vi"("error in"=w1795, "float32 argument"=w1796) -> ("error out"=w1792:errorcluster, "float32 data"=w1789:sgl)  [unwired: 8 in]
                    }
                    frame "/D48" {
                      n300 = call <vilib>:"Parse Message.vi"("error in"=w1804, "message"=w1805) -> ("error out"=w1806:errorcluster, "arguments"=w1808:T5[])  [unwired: 7 in, 1 out]
                      n301 = Index Array(array=w1808) -> (element=w1807:T5)  [unwired: 1 in]
                      n302 = call-poly <vilib>:"Argument to Data.vi"("error in"=w1806, "float32 argument"=w1807) -> ("error out"=w1803:errorcluster, "float32 data"=w1800:sgl)  [unwired: 8 in]
                      n303 = case shown="True" "OscBool" {
                        tunnel: [0 48] -> w1802
                        frame False {
                        }
                        frame True {
                        }
                      }
                    }
                    frame "/D49" {
                      n304 = local read "OscBool"() -> (w1812:bool)
                      n305 = case shown="True" w1812 {
                        tunnel: [0 49] -> w1813
                        frame False {
                        }
                        frame True {
                        }
                      }
                      n306 = call <vilib>:"Parse Message.vi"("error in"=w1815, "message"=w1816) -> ("error out"=w1819:errorcluster, "arguments"=w1817:T5[])  [unwired: 7 in, 1 out]
                      n307 = Index Array(array=w1817) -> (element=w1818:T5)  [unwired: 1 in]
                      n308 = call-poly <vilib>:"Argument to Data.vi"("error in"=w1819, "float32 argument"=w1818) -> ("error out"=w1814:errorcluster, "float32 data"=w1811:sgl)  [unwired: 8 in]
                    }
                    frame "/D50" {
                      n309 = local read "OscBool"() -> (w1823:bool)
                      n310 = call <vilib>:"Parse Message.vi"("error in"=w1825, "message"=w1826) -> ("error out"=w1828:errorcluster, "arguments"=w1830:T5[])  [unwired: 7 in, 1 out]
                      n311 = case shown="True" w1823 {
                        tunnel: [0 50] -> w1824
                        frame False {
                        }
                        frame True {
                        }
                      }
                      n312 = Index Array(array=w1830) -> (element=w1829:T5)  [unwired: 1 in]
                      n313 = call-poly <vilib>:"Argument to Data.vi"("error in"=w1828, "float32 argument"=w1829) -> ("error out"=w1827:errorcluster, "float32 data"=w1822:sgl)  [unwired: 8 in]
                    }
                    frame "/D51" {
                      n314 = local read "OscBool"() -> (w1834:bool)
                      n315 = case shown="True" w1834 {
                        tunnel: [0 51] -> w1835
                        frame False {
                        }
                        frame True {
                        }
                      }
                      n316 = call <vilib>:"Parse Message.vi"("error in"=w1836, "message"=w1837) -> ("error out"=w1841:errorcluster, "arguments"=w1839:T5[])  [unwired: 7 in, 1 out]
                      n317 = Index Array(array=w1839) -> (element=w1840:T5)  [unwired: 1 in]
                      n318 = call-poly <vilib>:"Argument to Data.vi"("error in"=w1841, "float32 argument"=w1840) -> ("error out"=w1838:errorcluster, "float32 data"=w1833:sgl)  [unwired: 8 in]
                    }
                    frame "/D52" {
                      n319 = local read "OscBool"() -> (w1845:bool)
                      n320 = call <vilib>:"Parse Message.vi"("error in"=w1848, "message"=w1847) -> ("error out"=w1852:errorcluster, "arguments"=w1850:T5[])  [unwired: 7 in, 1 out]
                      n321 = case shown="True" w1845 {
                        tunnel: [0 52] -> w1846
                        frame False {
                        }
                        frame True {
                        }
                      }
                      n322 = Index Array(array=w1850) -> (element=w1851:T5)  [unwired: 1 in]
                      n323 = call-poly <vilib>:"Argument to Data.vi"("error in"=w1852, "float32 argument"=w1851) -> ("error out"=w1849:errorcluster, "float32 data"=w1844:sgl)  [unwired: 8 in]
                    }
                    frame "/D53" {
                      n324 = local read "OscBool"() -> (w1856:bool)
                      n325 = call <vilib>:"Parse Message.vi"("error in"=w1858, "message"=w1859) -> ("error out"=w1863:errorcluster, "arguments"=w1861:T5[])  [unwired: 7 in, 1 out]
                      n326 = case shown="True" w1856 {
                        tunnel: [0 53] -> w1857
                        frame False {
                        }
                        frame True {
                        }
                      }
                      n327 = Index Array(array=w1861) -> (element=w1862:T5)  [unwired: 1 in]
                      n328 = call-poly <vilib>:"Argument to Data.vi"("error in"=w1863, "float32 argument"=w1862) -> ("error out"=w1860:errorcluster, "float32 data"=w1855:sgl)  [unwired: 8 in]
                    }
                    frame "/D54" {
                      n329 = local read "OscBool"() -> (w1867:bool)
                      n330 = case shown="True" w1867 {
                        tunnel: [0 54] -> w1868
                        frame False {
                        }
                        frame True {
                        }
                      }
                      n331 = call <vilib>:"Parse Message.vi"("error in"=w1869, "message"=w1870) -> ("error out"=w1872:errorcluster, "arguments"=w1874:T5[])  [unwired: 7 in, 1 out]
                      n332 = Index Array(array=w1874) -> (element=w1873:T5)  [unwired: 1 in]
                      n333 = call-poly <vilib>:"Argument to Data.vi"("error in"=w1872, "float32 argument"=w1873) -> ("error out"=w1871:errorcluster, "float32 data"=w1866:sgl)  [unwired: 8 in]
                    }
                    frame "/D55" {
                      n334 = local read "OscBool"() -> (w1879:bool)
                      n335 = case shown="True" w1879 {
                        tunnel: [0 55] -> w1878
                        frame False {
                        }
                        frame True {
                        }
                      }
                      n336 = call <vilib>:"Parse Message.vi"("error in"=w1881, "message"=w1880) -> ("error out"=w1885:errorcluster, "arguments"=w1883:T5[])  [unwired: 7 in, 1 out]
                      n337 = Index Array(array=w1883) -> (element=w1884:T5)  [unwired: 1 in]
                      n338 = call-poly <vilib>:"Argument to Data.vi"("error in"=w1885, "float32 argument"=w1884) -> ("error out"=w1882:errorcluster, "float32 data"=w1877:sgl)  [unwired: 8 in]
                    }
                    frame "/D56" {
                      n339 = local read "OscBool"() -> (w1890:bool)
                      n340 = case shown="True" w1890 {
                        tunnel: [0 56] -> w1889
                        frame False {
                        }
                        frame True {
                        }
                      }
                      n341 = call <vilib>:"Parse Message.vi"("error in"=w1891, "message"=w1892) -> ("error out"=w1894:errorcluster, "arguments"=w1896:T5[])  [unwired: 7 in, 1 out]
                      n342 = Index Array(array=w1896) -> (element=w1895:T5)  [unwired: 1 in]
                      n343 = call-poly <vilib>:"Argument to Data.vi"("error in"=w1894, "float32 argument"=w1895) -> ("error out"=w1893:errorcluster, "float32 data"=w1888:sgl)  [unwired: 8 in]
                    }
                    frame "/D57" {
                      n344 = local read "OscBool"() -> (w1901:bool)
                      n345 = case shown="True" w1901 {
                        tunnel: [0 57] -> w1900
                        frame False {
                        }
                        frame True {
                        }
                      }
                      n346 = call <vilib>:"Parse Message.vi"("error in"=w1902, "message"=w1903) -> ("error out"=w1907:errorcluster, "arguments"=w1905:T5[])  [unwired: 7 in, 1 out]
                      n347 = Index Array(array=w1905) -> (element=w1906:T5)  [unwired: 1 in]
                      n348 = call-poly <vilib>:"Argument to Data.vi"("error in"=w1907, "float32 argument"=w1906) -> ("error out"=w1904:errorcluster, "float32 data"=w1899:sgl)  [unwired: 8 in]
                    }
                    frame "/D58" {
                      n349 = local read "OscBool"() -> (w1912:bool)
                      n350 = case shown="True" w1912 {
                        tunnel: [0 58] -> w1911
                        frame False {
                        }
                        frame True {
                        }
                      }
                      n351 = call <vilib>:"Parse Message.vi"("error in"=w1913, "message"=w1914) -> ("error out"=w1918:errorcluster, "arguments"=w1916:T5[])  [unwired: 7 in, 1 out]
                      n352 = Index Array(array=w1916) -> (element=w1917:T5)  [unwired: 1 in]
                      n353 = call-poly <vilib>:"Argument to Data.vi"("error in"=w1918, "float32 argument"=w1917) -> ("error out"=w1915:errorcluster, "float32 data"=w1910:sgl)  [unwired: 8 in]
                    }
                    frame "/D59" {
                      n354 = call <vilib>:"Parse Message.vi"("error in"=w1923, "message"=w1924) -> ("error out"=w1928:errorcluster, "arguments"=w1926:T5[])  [unwired: 7 in, 1 out]
                      n355 = Index Array(array=w1926) -> (element=w1927:T5)  [unwired: 1 in]
                      n356 = call-poly <vilib>:"Argument to Data.vi"("error in"=w1928, "float32 argument"=w1927) -> ("error out"=w1925:errorcluster, "float32 data"=w1921:sgl)  [unwired: 8 in]
                    }
                    frame "/D60" {
                      n357 = call <vilib>:"Parse Message.vi"("error in"=w1931, "message"=w1932) -> ("error out"=w1936:errorcluster, "arguments"=w1934:T5[])  [unwired: 7 in, 1 out]
                      n358 = Index Array(array=w1934) -> (element=w1935:T5)  [unwired: 1 in]
                      n359 = call-poly <vilib>:"Argument to Data.vi"("error in"=w1936, "float32 argument"=w1935) -> ("error out"=w1933:errorcluster, "float32 data"=w1929:sgl)  [unwired: 8 in]
                    }
                    frame "/D61" {
                      n360 = call <vilib>:"Parse Message.vi"("error in"=w1939, "message"=w1940) -> ("error out"=w1944:errorcluster, "arguments"=w1942:T5[])  [unwired: 7 in, 1 out]
                      n361 = Index Array(array=w1942) -> (element=w1943:T5)  [unwired: 1 in]
                      n362 = call-poly <vilib>:"Argument to Data.vi"("error in"=w1944, "float32 argument"=w1943) -> ("error out"=w1941:errorcluster, "float32 data"=w1938:sgl)  [unwired: 8 in]
                    }
                    frame "/D62" {
                      n363 = call <vilib>:"Parse Message.vi"("error in"=w1947, "message"=w1948) -> ("error out"=w1952:errorcluster, "arguments"=w1950:T5[])  [unwired: 7 in, 1 out]
                      n364 = Index Array(array=w1950) -> (element=w1951:T5)  [unwired: 1 in]
                      n365 = call-poly <vilib>:"Argument to Data.vi"("error in"=w1952, "float32 argument"=w1951) -> ("error out"=w1949:errorcluster, "float32 data"=w1946:sgl)  [unwired: 8 in]
                    }
                    frame "/D63" {
                      n366 = call <vilib>:"Parse Message.vi"("error in"=w1955, "message"=w1956) -> ("error out"=w1960:errorcluster, "arguments"=w1958:T5[])  [unwired: 7 in, 1 out]
                      n367 = Index Array(array=w1958) -> (element=w1959:T5)  [unwired: 1 in]
                      n368 = call-poly <vilib>:"Argument to Data.vi"("error in"=w1960, "float32 argument"=w1959) -> ("error out"=w1957:errorcluster, "float32 data"=w1954:sgl)  [unwired: 8 in]
                    }
                    frame "/D64" {
                      n369 = call <vilib>:"Parse Message.vi"("error in"=w1964, "message"=w1963) -> ("error out"=w1966:errorcluster, "arguments"=w1968:T5[])  [unwired: 7 in, 1 out]
                      n370 = Index Array(array=w1968) -> (element=w1967:T5)  [unwired: 1 in]
                      n371 = call-poly <vilib>:"Argument to Data.vi"("error in"=w1966, "float32 argument"=w1967) -> ("error out"=w1965:errorcluster, "float32 data"=w1961:sgl)  [unwired: 8 in]
                    }
                    frame "/MIDI" {
                      n372 = call <vilib>:"Parse Message.vi"("error in"=w1974, "message"=w1975) -> ("error out"=w1976:errorcluster, "arguments"=w1978:T5[])  [unwired: 7 in, 1 out]
                      n373 = Index Array(array=w1978) -> (element=w1977:T5)  [unwired: 1 in]
                      n374 = call-poly <vilib>:"Argument to Data.vi"("error in"=w1976, "float32 argument"=w1977) -> ("error out"=w1973:errorcluster, "float32 data"=w1969:sgl)  [unwired: 8 in]
                      n375 = Not Equal To 0?(x=w1969) -> (x != 0?=w1970:bool)
                      n376 = case shown="False" w1970 {
                        frame False {
                          n377 = local write "MidiBool"(FALSE ("MidiBool")) -> ()
                        }
                        frame True {
                          n378 = local write "MidiBool"(TRUE ("MidiBool")) -> ()
                        }
                      }
                    }
                    frame "/OSC" {
                      n379 = call <vilib>:"Parse Message.vi"("error in"=w1986, "message"=w1987) -> ("error out"=w1988:errorcluster, "arguments"=w1990:T5[])  [unwired: 7 in, 1 out]
                      n380 = Index Array(array=w1990) -> (element=w1989:T5)  [unwired: 1 in]
                      n381 = call-poly <vilib>:"Argument to Data.vi"("error in"=w1988, "float32 argument"=w1989) -> ("error out"=w1985:errorcluster, "float32 data"=w1981:sgl)  [unwired: 8 in]
                      n382 = Not Equal To 0?(x=w1981) -> (x != 0?=w1982:bool)
                      n383 = case shown="True" w1982 {
                        frame False {
                          n384 = local write "OscBool"(FALSE ("OscBool")) -> ()
                        }
                        frame True {
                          n385 = local write "OscBool"(TRUE ("OscBool")) -> ()
                        }
                      }
                    }
                    frame "/AllZero" {
                      n386 = call <vilib>:"Parse Message.vi"("error in"=w1998, "message"=w1996) -> ("error out"=w1999:errorcluster, "arguments"=w2001:T5[])  [unwired: 7 in, 1 out]
                      n387 = Index Array(array=w2001) -> (element=w2000:T5)  [unwired: 1 in]
                      n388 = call-poly <vilib>:"Argument to Data.vi"("error in"=w1999, "float32 argument"=w2000) -> ("error out"=w1997:errorcluster, "float32 data"=w1994:sgl)  [unwired: 8 in]
                      n389 = Not Equal To 0?(x=w1994) -> (x != 0?=w1993:bool)
                      n390 = case shown="True" w1993 {
                        tunnel: [0 65] -> w1995
                        frame False {
                        }
                        frame True {
                        }
                      }
                    }
                  }
                }
              }
              frame Error {
                # "There was no data available, so ignore error 56 (timed out)."
                n391 = Unbundle By Name(w2007) -> ("code"=w2008:i32)
                n392 = case shown="Default" w2008 {
                  tunnel: w2007 -> [w2009 _ _]
                  tunnel: [w2009 _ _] -> w2006
                  frame Default {
                  }
                  frame 1 {
                  }
                  frame 56 {
                  }
                }
              }
            }
            n393 = To Double Precision Float(number=w1260) -> (double precision float=w1259:dbl)
          }
        }
        n394 = disable-structure shown="Enabled" {
          disable-tunnel: w139 -> [_ w167]
          disable-tunnel: w140 -> [_ w166]
          disable-tunnel: w138 -> [_ w165]
          disable-tunnel: [w157 w164] -> w132
          disable-tunnel: [w156 w163] -> w131
          disable-tunnel: [_ w162] -> w130
          disable-tunnel: w129 -> [w157 w161]
          disable-tunnel: w128 -> [w156 w160]
          disable-tunnel: w127 -> [_ w159]
          frame Disabled {
          }
          frame Enabled {
            n395 = case shown="0" w166 {
              tunnel: w167 -> [_ w179]
              tunnel: w165 -> [_ w178]
              tunnel: [w170 w177] -> w164
              tunnel: [w169 w176] -> w163
              tunnel: [0 ("9401/Slot 3 Error Code") w175] -> w162
              tunnel: w159 -> [_ w174]
              tunnel: w161 -> [w170 w173]
              tunnel: w160 -> [w169 w172]
              tunnel: 800000.0 ("x") -> [_ w171]
              frame Default {
              }
              frame 0 {
                n396 = case shown="65" w179 {
                  tunnel: w178 -> [_ w185 w194 w203 w212 w221 w230 w239 w248 w257 w266 w275 w284 w293 w302 w311 w320 w330 w338 w348 w357 w368 w377 w386 w395 w401 w410 w419 w428 w437 w446 w455 w464 w473 w482 w491 w500 w509 w518 w527 w536 w545 w554 w564 w572 w581 w590 w599 w609 w617 w626 w635 w644 w653 w662 w671 w680 w689 w698 w707 w731 w755 w779 w803 w827 _]
                  tunnel: [w183 w193 w202 w211 w220 w229 w238 w247 w256 w265 w274 w283 w292 w301 w310 w319 w328 w337 w343 w352 w360 w369 w378 w387 w398 w409 w418 w427 w436 w445 w454 w463 w472 w481 w490 w499 w508 w517 w526 w534 w543 w552 w561 w570 w579 w588 w597 w606 w615 w624 w633 w642 w651 w660 w669 w678 w687 w696 w705 w714 w738 w762 w786 w810 w834 w856] -> w177
                  tunnel: [w182 w192 w201 w210 w219 w228 w237 w246 w255 w264 w273 w282 w291 w300 w309 w318 w327 w336 w342 w351 w361 w370 w379 w388 w397 w408 w417 w426 w435 w444 w453 w462 w471 w480 w489 w498 w507 w516 w525 w533 w542 w551 w560 w569 w578 w587 w596 w605 w614 w623 w632 w641 w650 w659 w668 w677 w686 w695 w704 w713 w737 w761 w785 w809 w833 w855] -> w176
                  tunnel: [w184 w191 w200 w209 w218 w227 w236 w245 w254 w263 w272 w281 w290 w299 w308 w317 w326 w335 w344 w353 w362 w371 w380 w389 w396 w407 w416 w425 w434 w443 w452 w461 w470 w479 w488 w497 w506 w515 w524 w535 w544 w553 w562 w571 w580 w589 w598 w607 w616 w625 w634 w643 w652 w661 w670 w679 w688 w697 w706 w712 w736 w760 w784 w808 w832 w854] -> w175
                  tunnel: w174 -> [_ w186 w195 w204 w213 w222 w231 w240 w249 w258 w267 w276 w285 w294 w303 w312 w321 w329 w339 w347 w356 w367 w376 w385 w394 w402 w411 w420 w429 w438 w447 w456 w465 w474 w483 w492 w501 w510 w519 w528 w537 w546 w555 w563 w573 w582 w591 w600 w608 w618 w627 w636 w645 w654 w663 w672 w681 w690 w699 _ _ _ _ _ _ _]
                  tunnel: w173 -> [w181 w190 w199 w208 w217 w226 w235 w244 w253 w262 w271 w280 w289 w298 w307 w316 w325 w332 w341 w350 w359 w366 w375 w384 w393 w406 w415 w424 w433 w442 w451 w460 w469 w478 w487 w496 w505 w514 w523 w532 w541 w550 w559 w568 w577 w586 w595 w604 w613 w622 w631 w640 w649 w658 w667 w676 w685 w694 w703 w711 w735 w759 w781 w805 w831 w852]
                  tunnel: w172 -> [w180 w189 w198 w207 w216 w225 w234 w243 w252 w261 w270 w279 w288 w297 w306 w315 w324 w331 w340 w349 w358 w365 w374 w383 w392 w405 w414 w423 w432 w441 w450 w459 w468 w477 w486 w495 w504 w513 w522 w531 w540 w549 w558 w567 w576 w585 w594 w603 w612 w621 w630 w639 w648 w657 w666 w675 w684 w693 w702 w710 w734 w758 w782 w806 w830 w853]
                  tunnel: w171 -> [_ _ _ _ _ _ _ _ _ _ _ _ _ _ _ _ _ _ _ _ _ _ _ _ _ _ _ _ _ _ _ _ _ _ _ _ _ _ _ _ _ _ _ _ _ _ _ _ _ _ _ _ _ _ _ _ _ _ _ w709 w733 w757 w783 w807 w829 _]
                  frame 0, Default {
                    n397 = xnode "Read/Write Control"("FPGA VI Reference In"=w181, "error in"=w180) -> ("FPGA VI Reference Out"=w183:refnum<k20>, "error out"=w182:errorcluster, "9401/Slot 3 Error Code"=w184:i32)
                  }
                  frame 1 {
                    n398 = Multiply(x=w185, y=w186) -> (x*y=w187:dbl)
                    n399 = To Long Integer(number=w187) -> (32bit integer=w188:i32)
                    n400 = xnode "Read/Write Control"("FPGA VI Reference In"=w190, "error in"=w189, "PWM Duty Cycle (Ticks) 1"=w188) -> ("FPGA VI Reference Out"=w193:refnum<k20>, "error out"=w192:errorcluster, "9401/Slot 3 Error Code"=w191:i32)
                    "/D1" <- w185
                  }
                  frame 2 {
                    n401 = Multiply(x=w194, y=w195) -> (x*y=w196:dbl)
                    n402 = To Long Integer(number=w196) -> (32bit integer=w197:i32)
                    n403 = xnode "Read/Write Control"("FPGA VI Reference In"=w199, "error in"=w198, "PWM Duty Cycle (Ticks) 2"=w197) -> ("FPGA VI Reference Out"=w202:refnum<k20>, "error out"=w201:errorcluster, "9401/Slot 3 Error Code"=w200:i32)
                    "/D2" <- w194
                  }
                  frame 3 {
                    n404 = Multiply(x=w203, y=w204) -> (x*y=w205:dbl)
                    n405 = To Long Integer(number=w205) -> (32bit integer=w206:i32)
                    n406 = xnode "Read/Write Control"("FPGA VI Reference In"=w208, "error in"=w207, "PWM Duty Cycle (Ticks) 3"=w206) -> ("FPGA VI Reference Out"=w211:refnum<k20>, "error out"=w210:errorcluster, "9401/Slot 3 Error Code"=w209:i32)
                    "/D3" <- w203
                  }
                  frame 4 {
                    n407 = Multiply(x=w212, y=w213) -> (x*y=w214:dbl)
                    n408 = To Long Integer(number=w214) -> (32bit integer=w215:i32)
                    n409 = xnode "Read/Write Control"("FPGA VI Reference In"=w217, "error in"=w216, "PWM Duty Cycle (Ticks) 4"=w215) -> ("FPGA VI Reference Out"=w220:refnum<k20>, "error out"=w219:errorcluster, "9401/Slot 3 Error Code"=w218:i32)
                    "/D4" <- w212
                  }
                  frame 5 {
                    n410 = Multiply(x=w221, y=w222) -> (x*y=w223:dbl)
                    n411 = To Long Integer(number=w223) -> (32bit integer=w224:i32)
                    n412 = xnode "Read/Write Control"("FPGA VI Reference In"=w226, "error in"=w225, "PWM Duty Cycle (Ticks) 5"=w224) -> ("FPGA VI Reference Out"=w229:refnum<k20>, "error out"=w228:errorcluster, "9401/Slot 3 Error Code"=w227:i32)
                    "/D5" <- w221
                  }
                  frame 6 {
                    n413 = Multiply(x=w230, y=w231) -> (x*y=w232:dbl)
                    n414 = To Long Integer(number=w232) -> (32bit integer=w233:i32)
                    n415 = xnode "Read/Write Control"("FPGA VI Reference In"=w235, "error in"=w234, "PWM Duty Cycle (Ticks) 6"=w233) -> ("FPGA VI Reference Out"=w238:refnum<k20>, "error out"=w237:errorcluster, "9401/Slot 3 Error Code"=w236:i32)
                    "/D6" <- w230
                  }
                  frame 7 {
                    n416 = Multiply(x=w239, y=w240) -> (x*y=w241:dbl)
                    n417 = To Long Integer(number=w241) -> (32bit integer=w242:i32)
                    n418 = xnode "Read/Write Control"("FPGA VI Reference In"=w244, "error in"=w243, "PWM Duty Cycle (Ticks) 7"=w242) -> ("FPGA VI Reference Out"=w247:refnum<k20>, "error out"=w246:errorcluster, "9401/Slot 3 Error Code"=w245:i32)
                    "/D7" <- w239
                  }
                  frame 8 {
                    n419 = Multiply(x=w248, y=w249) -> (x*y=w250:dbl)
                    n420 = To Long Integer(number=w250) -> (32bit integer=w251:i32)
                    n421 = xnode "Read/Write Control"("FPGA VI Reference In"=w253, "error in"=w252, "PWM Duty Cycle (Ticks) 8"=w251) -> ("FPGA VI Reference Out"=w256:refnum<k20>, "error out"=w255:errorcluster, "9401/Slot 3 Error Code"=w254:i32)
                    "/D8" <- w248
                  }
                  frame 9 {
                    n422 = Multiply(x=w257, y=w258) -> (x*y=w259:dbl)
                    n423 = To Long Integer(number=w259) -> (32bit integer=w260:i32)
                    n424 = xnode "Read/Write Control"("FPGA VI Reference In"=w262, "error in"=w261, "PWM Duty Cycle (Ticks) 9"=w260) -> ("FPGA VI Reference Out"=w265:refnum<k20>, "error out"=w264:errorcluster, "9401/Slot 3 Error Code"=w263:i32)
                    "/D9" <- w257
                  }
                  frame 10 {
                    n425 = Multiply(x=w266, y=w267) -> (x*y=w268:dbl)
                    n426 = To Long Integer(number=w268) -> (32bit integer=w269:i32)
                    n427 = xnode "Read/Write Control"("FPGA VI Reference In"=w271, "error in"=w270, "PWM Duty Cycle (Ticks) 10"=w269) -> ("FPGA VI Reference Out"=w274:refnum<k20>, "error out"=w273:errorcluster, "9401/Slot 3 Error Code"=w272:i32)
                    "/D10" <- w266
                  }
                  frame 11 {
                    n428 = Multiply(x=w275, y=w276) -> (x*y=w277:dbl)
                    n429 = To Long Integer(number=w277) -> (32bit integer=w278:i32)
                    n430 = xnode "Read/Write Control"("FPGA VI Reference In"=w280, "error in"=w279, "PWM Duty Cycle (Ticks) 11"=w278) -> ("FPGA VI Reference Out"=w283:refnum<k20>, "error out"=w282:errorcluster, "9401/Slot 3 Error Code"=w281:i32)
                    "/D11" <- w275
                  }
                  frame 12 {
                    n431 = Multiply(x=w284, y=w285) -> (x*y=w286:dbl)
                    n432 = To Long Integer(number=w286) -> (32bit integer=w287:i32)
                    n433 = xnode "Read/Write Control"("FPGA VI Reference In"=w289, "error in"=w288, "PWM Duty Cycle (Ticks) 12"=w287) -> ("FPGA VI Reference Out"=w292:refnum<k20>, "error out"=w291:errorcluster, "9401/Slot 3 Error Code"=w290:i32)
                    "/D12" <- w284
                  }
                  frame 13 {
                    n434 = Multiply(x=w293, y=w294) -> (x*y=w295:dbl)
                    n435 = To Long Integer(number=w295) -> (32bit integer=w296:i32)
                    n436 = xnode "Read/Write Control"("FPGA VI Reference In"=w298, "error in"=w297, "PWM Duty Cycle (Ticks) 13"=w296) -> ("FPGA VI Reference Out"=w301:refnum<k20>, "error out"=w300:errorcluster, "9401/Slot 3 Error Code"=w299:i32)
                    "/D13" <- w293
                  }
                  frame 14 {
                    n437 = Multiply(x=w302, y=w303) -> (x*y=w304:dbl)
                    n438 = To Long Integer(number=w304) -> (32bit integer=w305:i32)
                    n439 = xnode "Read/Write Control"("FPGA VI Reference In"=w307, "error in"=w306, "PWM Duty Cycle (Ticks) 14"=w305) -> ("FPGA VI Reference Out"=w310:refnum<k20>, "error out"=w309:errorcluster, "9401/Slot 3 Error Code"=w308:i32)
                    "/D14" <- w302
                  }
                  frame 15 {
                    n440 = Multiply(x=w311, y=w312) -> (x*y=w313:dbl)
                    n441 = To Long Integer(number=w313) -> (32bit integer=w314:i32)
                    n442 = xnode "Read/Write Control"("FPGA VI Reference In"=w316, "error in"=w315, "PWM Duty Cycle (Ticks) 15"=w314) -> ("FPGA VI Reference Out"=w319:refnum<k20>, "error out"=w318:errorcluster, "9401/Slot 3 Error Code"=w317:i32)
                    "/D15" <- w311
                  }
                  frame 16 {
                    n443 = Multiply(x=w320, y=w321) -> (x*y=w322:dbl)
                    n444 = To Long Integer(number=w322) -> (32bit integer=w323:i32)
                    n445 = xnode "Read/Write Control"("FPGA VI Reference In"=w325, "error in"=w324, "PWM Duty Cycle (Ticks) 16"=w323) -> ("FPGA VI Reference Out"=w328:refnum<k20>, "error out"=w327:errorcluster, "9401/Slot 3 Error Code"=w326:i32)
                    "/D16" <- w320
                  }
                  frame 17 {
                    n446 = Multiply(x=w330, y=w329) -> (x*y=w334:dbl)
                    n447 = To Long Integer(number=w334) -> (32bit integer=w333:i32)
                    n448 = xnode "Read/Write Control"("FPGA VI Reference In"=w332, "error in"=w331, "PWM Duty Cycle (Ticks) 17"=w333) -> ("FPGA VI Reference Out"=w337:refnum<k20>, "error out"=w336:errorcluster, "9401/Slot 3 Error Code"=w335:i32)
                    "/D17" <- w330
                  }
                  frame 18 {
                    n449 = Multiply(x=w338, y=w339) -> (x*y=w345:dbl)
                    n450 = To Long Integer(number=w345) -> (32bit integer=w346:i32)
                    n451 = xnode "Read/Write Control"("FPGA VI Reference In"=w341, "error in"=w340, "PWM Duty Cycle (Ticks) 18"=w346) -> ("FPGA VI Reference Out"=w343:refnum<k20>, "error out"=w342:errorcluster, "9401/Slot 3 Error Code"=w344:i32)
                    "/D18" <- w338
                  }
                  frame 19 {
                    n452 = Multiply(x=w348, y=w347) -> (x*y=w355:dbl)
                    n453 = To Long Integer(number=w355) -> (32bit integer=w354:i32)
                    n454 = xnode "Read/Write Control"("FPGA VI Reference In"=w350, "error in"=w349, "PWM Duty Cycle (Ticks) 19"=w354) -> ("FPGA VI Reference Out"=w352:refnum<k20>, "error out"=w351:errorcluster, "9401/Slot 3 Error Code"=w353:i32)
                    "/D19" <- w348
                  }
                  frame 20 {
                    n455 = Multiply(x=w357, y=w356) -> (x*y=w363:dbl)
                    n456 = To Long Integer(number=w363) -> (32bit integer=w364:i32)
                    n457 = xnode "Read/Write Control"("FPGA VI Reference In"=w359, "error in"=w358, "PWM Duty Cycle (Ticks) 20"=w364) -> ("FPGA VI Reference Out"=w360:refnum<k20>, "error out"=w361:errorcluster, "9401/Slot 3 Error Code"=w362:i32)
                    "/D20" <- w357
                  }
                  frame 21 {
                    n458 = Multiply(x=w368, y=w367) -> (x*y=w373:dbl)
                    n459 = To Long Integer(number=w373) -> (32bit integer=w372:i32)
                    n460 = xnode "Read/Write Control"("FPGA VI Reference In"=w366, "error in"=w365, "PWM Duty Cycle (Ticks) 21"=w372) -> ("FPGA VI Reference Out"=w369:refnum<k20>, "error out"=w370:errorcluster, "9401/Slot 3 Error Code"=w371:i32)
                    "/D21" <- w368
                  }
                  frame 22 {
                    n461 = Multiply(x=w377, y=w376) -> (x*y=w382:dbl)
                    n462 = To Long Integer(number=w382) -> (32bit integer=w381:i32)
                    n463 = xnode "Read/Write Control"("FPGA VI Reference In"=w375, "error in"=w374, "PWM Duty Cycle (Ticks) 22"=w381) -> ("FPGA VI Reference Out"=w378:refnum<k20>, "error out"=w379:errorcluster, "9401/Slot 3 Error Code"=w380:i32)
                    "/D22" <- w377
                  }
                  frame 23 {
                    n464 = Multiply(x=w386, y=w385) -> (x*y=w391:dbl)
                    n465 = To Long Integer(number=w391) -> (32bit integer=w390:i32)
                    n466 = xnode "Read/Write Control"("FPGA VI Reference In"=w384, "error in"=w383, "PWM Duty Cycle (Ticks) 23"=w390) -> ("FPGA VI Reference Out"=w387:refnum<k20>, "error out"=w388:errorcluster, "9401/Slot 3 Error Code"=w389:i32)
                    "/D23" <- w386
                  }
                  frame 24 {
                    n467 = Multiply(x=w395, y=w394) -> (x*y=w400:dbl)
                    n468 = To Long Integer(number=w400) -> (32bit integer=w399:i32)
                    n469 = xnode "Read/Write Control"("FPGA VI Reference In"=w393, "error in"=w392, "PWM Duty Cycle (Ticks) 24"=w399) -> ("FPGA VI Reference Out"=w398:refnum<k20>, "error out"=w397:errorcluster, "9401/Slot 3 Error Code"=w396:i32)
                    "/D24" <- w395
                  }
                  frame 25 {
                    n470 = Multiply(x=w401, y=w402) -> (x*y=w404:dbl)
                    n471 = To Long Integer(number=w404) -> (32bit integer=w403:i32)
                    n472 = xnode "Read/Write Control"("FPGA VI Reference In"=w406, "error in"=w405, "PWM Duty Cycle (Ticks) 25"=w403) -> ("FPGA VI Reference Out"=w409:refnum<k20>, "error out"=w408:errorcluster, "9401/Slot 3 Error Code"=w407:i32)
                    "/D25" <- w401
                  }
                  frame 26 {
                    n473 = Multiply(x=w410, y=w411) -> (x*y=w413:dbl)
                    n474 = To Long Integer(number=w413) -> (32bit integer=w412:i32)
                    n475 = xnode "Read/Write Control"("FPGA VI Reference In"=w415, "error in"=w414, "PWM Duty Cycle (Ticks) 26"=w412) -> ("FPGA VI Reference Out"=w418:refnum<k20>, "error out"=w417:errorcluster, "9401/Slot 3 Error Code"=w416:i32)
                    "/D26" <- w410
                  }
                  frame 27 {
                    n476 = Multiply(x=w419, y=w420) -> (x*y=w422:dbl)
                    n477 = To Long Integer(number=w422) -> (32bit integer=w421:i32)
                    n478 = xnode "Read/Write Control"("FPGA VI Reference In"=w424, "error in"=w423, "PWM Duty Cycle (Ticks) 27"=w421) -> ("FPGA VI Reference Out"=w427:refnum<k20>, "error out"=w426:errorcluster, "9401/Slot 3 Error Code"=w425:i32)
                    "/D27" <- w419
                  }
                  frame 28 {
                    n479 = Multiply(x=w428, y=w429) -> (x*y=w431:dbl)
                    n480 = To Long Integer(number=w431) -> (32bit integer=w430:i32)
                    n481 = xnode "Read/Write Control"("FPGA VI Reference In"=w433, "error in"=w432, "PWM Duty Cycle (Ticks) 28"=w430) -> ("FPGA VI Reference Out"=w436:refnum<k20>, "error out"=w435:errorcluster, "9401/Slot 3 Error Code"=w434:i32)
                    "/D28" <- w428
                  }
                  frame 29 {
                    n482 = Multiply(x=w437, y=w438) -> (x*y=w440:dbl)
                    n483 = To Long Integer(number=w440) -> (32bit integer=w439:i32)
                    n484 = xnode "Read/Write Control"("FPGA VI Reference In"=w442, "error in"=w441, "PWM Duty Cycle (Ticks) 29"=w439) -> ("FPGA VI Reference Out"=w445:refnum<k20>, "error out"=w444:errorcluster, "9401/Slot 3 Error Code"=w443:i32)
                    "/D29" <- w437
                  }
                  frame 30 {
                    n485 = Multiply(x=w446, y=w447) -> (x*y=w449:dbl)
                    n486 = To Long Integer(number=w449) -> (32bit integer=w448:i32)
                    n487 = xnode "Read/Write Control"("FPGA VI Reference In"=w451, "error in"=w450, "PWM Duty Cycle (Ticks) 30"=w448) -> ("FPGA VI Reference Out"=w454:refnum<k20>, "error out"=w453:errorcluster, "9401/Slot 3 Error Code"=w452:i32)
                    "/D30" <- w446
                  }
                  frame 31 {
                    n488 = Multiply(x=w455, y=w456) -> (x*y=w458:dbl)
                    n489 = To Long Integer(number=w458) -> (32bit integer=w457:i32)
                    n490 = xnode "Read/Write Control"("FPGA VI Reference In"=w460, "error in"=w459, "PWM Duty Cycle (Ticks) 31"=w457) -> ("FPGA VI Reference Out"=w463:refnum<k20>, "error out"=w462:errorcluster, "9401/Slot 3 Error Code"=w461:i32)
                    "/D31" <- w455
                  }
                  frame 32 {
                    n491 = Multiply(x=w464, y=w465) -> (x*y=w467:dbl)
                    n492 = To Long Integer(number=w467) -> (32bit integer=w466:i32)
                    n493 = xnode "Read/Write Control"("FPGA VI Reference In"=w469, "error in"=w468, "PWM Duty Cycle (Ticks) 32"=w466) -> ("FPGA VI Reference Out"=w472:refnum<k20>, "error out"=w471:errorcluster, "9401/Slot 3 Error Code"=w470:i32)
                    "/D32" <- w464
                  }
                  frame 33 {
                    n494 = Multiply(x=w473, y=w474) -> (x*y=w476:dbl)
                    n495 = To Long Integer(number=w476) -> (32bit integer=w475:i32)
                    n496 = xnode "Read/Write Control"("FPGA VI Reference In"=w478, "error in"=w477, "PWM Duty Cycle (Ticks) 33"=w475) -> ("FPGA VI Reference Out"=w481:refnum<k20>, "error out"=w480:errorcluster, "9401/Slot 3 Error Code"=w479:i32)
                    "/D33" <- w473
                  }
                  frame 34 {
                    n497 = Multiply(x=w482, y=w483) -> (x*y=w485:dbl)
                    n498 = To Long Integer(number=w485) -> (32bit integer=w484:i32)
                    n499 = xnode "Read/Write Control"("FPGA VI Reference In"=w487, "error in"=w486, "PWM Duty Cycle (Ticks) 34"=w484) -> ("FPGA VI Reference Out"=w490:refnum<k20>, "error out"=w489:errorcluster, "9401/Slot 3 Error Code"=w488:i32)
                    "/D34" <- w482
                  }
                  frame 35 {
                    n500 = Multiply(x=w491, y=w492) -> (x*y=w494:dbl)
                    n501 = To Long Integer(number=w494) -> (32bit integer=w493:i32)
                    n502 = xnode "Read/Write Control"("FPGA VI Reference In"=w496, "error in"=w495, "PWM Duty Cycle (Ticks) 35"=w493) -> ("FPGA VI Reference Out"=w499:refnum<k20>, "error out"=w498:errorcluster, "9401/Slot 3 Error Code"=w497:i32)
                    "/D35" <- w491
                  }
                  frame 36 {
                    n503 = Multiply(x=w500, y=w501) -> (x*y=w503:dbl)
                    n504 = To Long Integer(number=w503) -> (32bit integer=w502:i32)
                    n505 = xnode "Read/Write Control"("FPGA VI Reference In"=w505, "error in"=w504, "PWM Duty Cycle (Ticks) 36"=w502) -> ("FPGA VI Reference Out"=w508:refnum<k20>, "error out"=w507:errorcluster, "9401/Slot 3 Error Code"=w506:i32)
                    "/D36" <- w500
                  }
                  frame 37 {
                    n506 = Multiply(x=w509, y=w510) -> (x*y=w512:dbl)
                    n507 = To Long Integer(number=w512) -> (32bit integer=w511:i32)
                    n508 = xnode "Read/Write Control"("FPGA VI Reference In"=w514, "error in"=w513, "PWM Duty Cycle (Ticks) 37"=w511) -> ("FPGA VI Reference Out"=w517:refnum<k20>, "error out"=w516:errorcluster, "9401/Slot 3 Error Code"=w515:i32)
                    "/D37" <- w509
                  }
                  frame 38 {
                    n509 = Multiply(x=w518, y=w519) -> (x*y=w521:dbl)
                    n510 = To Long Integer(number=w521) -> (32bit integer=w520:i32)
                    n511 = xnode "Read/Write Control"("FPGA VI Reference In"=w523, "error in"=w522, "PWM Duty Cycle (Ticks) 38"=w520) -> ("FPGA VI Reference Out"=w526:refnum<k20>, "error out"=w525:errorcluster, "9401/Slot 3 Error Code"=w524:i32)
                    "/D38" <- w518
                  }
                  frame 39 {
                    n512 = Multiply(x=w527, y=w528) -> (x*y=w530:dbl)
                    n513 = To Long Integer(number=w530) -> (32bit integer=w529:i32)
                    n514 = xnode "Read/Write Control"("FPGA VI Reference In"=w532, "error in"=w531, "PWM Duty Cycle (Ticks) 39"=w529) -> ("FPGA VI Reference Out"=w534:refnum<k20>, "error out"=w533:errorcluster, "9401/Slot 3 Error Code"=w535:i32)
                    "/D39" <- w527
                  }
                  frame 40 {
                    n515 = Multiply(x=w536, y=w537) -> (x*y=w539:dbl)
                    n516 = To Long Integer(number=w539) -> (32bit integer=w538:i32)
                    n517 = xnode "Read/Write Control"("FPGA VI Reference In"=w541, "error in"=w540, "PWM Duty Cycle (Ticks) 40"=w538) -> ("FPGA VI Reference Out"=w543:refnum<k20>, "error out"=w542:errorcluster, "9401/Slot 3 Error Code"=w544:i32)
                    "/D40" <- w536
                  }
                  frame 41 {
                    n518 = Multiply(x=w545, y=w546) -> (x*y=w548:dbl)
                    n519 = To Long Integer(number=w548) -> (32bit integer=w547:i32)
                    n520 = xnode "Read/Write Control"("FPGA VI Reference In"=w550, "error in"=w549, "PWM Duty Cycle (Ticks) 41"=w547) -> ("FPGA VI Reference Out"=w552:refnum<k20>, "error out"=w551:errorcluster, "9401/Slot 3 Error Code"=w553:i32)
                    "/D41" <- w545
                  }
                  frame 42 {
                    n521 = Multiply(x=w554, y=w555) -> (x*y=w557:dbl)
                    n522 = To Long Integer(number=w557) -> (32bit integer=w556:i32)
                    n523 = xnode "Read/Write Control"("FPGA VI Reference In"=w559, "error in"=w558, "PWM Duty Cycle (Ticks) 42"=w556) -> ("FPGA VI Reference Out"=w561:refnum<k20>, "error out"=w560:errorcluster, "9401/Slot 3 Error Code"=w562:i32)
                    "/D42" <- w554
                  }
                  frame 43 {
                    n524 = Multiply(x=w564, y=w563) -> (x*y=w566:dbl)
                    n525 = To Long Integer(number=w566) -> (32bit integer=w565:i32)
                    n526 = xnode "Read/Write Control"("FPGA VI Reference In"=w568, "error in"=w567, "PWM Duty Cycle (Ticks) 43"=w565) -> ("FPGA VI Reference Out"=w570:refnum<k20>, "error out"=w569:errorcluster, "9401/Slot 3 Error Code"=w571:i32)
                    "/D43" <- w564
                  }
                  frame 44 {
                    n527 = Multiply(x=w572, y=w573) -> (x*y=w575:dbl)
                    n528 = To Long Integer(number=w575) -> (32bit integer=w574:i32)
                    n529 = xnode "Read/Write Control"("FPGA VI Reference In"=w577, "error in"=w576, "PWM Duty Cycle (Ticks) 44"=w574) -> ("FPGA VI Reference Out"=w579:refnum<k20>, "error out"=w578:errorcluster, "9401/Slot 3 Error Code"=w580:i32)
                    "/D44" <- w572
                  }
                  frame 45 {
                    n530 = Multiply(x=w581, y=w582) -> (x*y=w584:dbl)
                    n531 = To Long Integer(number=w584) -> (32bit integer=w583:i32)
                    n532 = xnode "Read/Write Control"("FPGA VI Reference In"=w586, "error in"=w585, "PWM Duty Cycle (Ticks) 45"=w583) -> ("FPGA VI Reference Out"=w588:refnum<k20>, "error out"=w587:errorcluster, "9401/Slot 3 Error Code"=w589:i32)
                    "/D45" <- w581
                  }
                  frame 46 {
                    n533 = Multiply(x=w590, y=w591) -> (x*y=w593:dbl)
                    n534 = To Long Integer(number=w593) -> (32bit integer=w592:i32)
                    n535 = xnode "Read/Write Control"("FPGA VI Reference In"=w595, "error in"=w594, "PWM Duty Cycle (Ticks) 46"=w592) -> ("FPGA VI Reference Out"=w597:refnum<k20>, "error out"=w596:errorcluster, "9401/Slot 3 Error Code"=w598:i32)
                    "/D46" <- w590
                  }
                  frame 47 {
                    n536 = Multiply(x=w599, y=w600) -> (x*y=w602:dbl)
                    n537 = To Long Integer(number=w602) -> (32bit integer=w601:i32)
                    n538 = xnode "Read/Write Control"("FPGA VI Reference In"=w604, "error in"=w603, "PWM Duty Cycle (Ticks) 47"=w601) -> ("FPGA VI Reference Out"=w606:refnum<k20>, "error out"=w605:errorcluster, "9401/Slot 3 Error Code"=w607:i32)
                    "/D47" <- w599
                  }
                  frame 48 {
                    n539 = Multiply(x=w609, y=w608) -> (x*y=w611:dbl)
                    n540 = To Long Integer(number=w611) -> (32bit integer=w610:i32)
                    n541 = xnode "Read/Write Control"("FPGA VI Reference In"=w613, "error in"=w612, "PWM Duty Cycle (Ticks) 48"=w610) -> ("FPGA VI Reference Out"=w615:refnum<k20>, "error out"=w614:errorcluster, "9401/Slot 3 Error Code"=w616:i32)
                    "/D48" <- w609
                  }
                  frame 49 {
                    n542 = Multiply(x=w617, y=w618) -> (x*y=w620:dbl)
                    n543 = To Long Integer(number=w620) -> (32bit integer=w619:i32)
                    n544 = xnode "Read/Write Control"("FPGA VI Reference In"=w622, "error in"=w621, "PWM Duty Cycle (Ticks) 49"=w619) -> ("FPGA VI Reference Out"=w624:refnum<k20>, "error out"=w623:errorcluster, "9401/Slot 3 Error Code"=w625:i32)
                    "/D49" <- w617
                  }
                  frame 50 {
                    n545 = Multiply(x=w626, y=w627) -> (x*y=w629:dbl)
                    n546 = To Long Integer(number=w629) -> (32bit integer=w628:i32)
                    n547 = xnode "Read/Write Control"("FPGA VI Reference In"=w631, "error in"=w630, "PWM Duty Cycle (Ticks) 50"=w628) -> ("FPGA VI Reference Out"=w633:refnum<k20>, "error out"=w632:errorcluster, "9401/Slot 3 Error Code"=w634:i32)
                    "/D50" <- w626
                  }
                  frame 51 {
                    n548 = Multiply(x=w635, y=w636) -> (x*y=w638:dbl)
                    n549 = To Long Integer(number=w638) -> (32bit integer=w637:i32)
                    n550 = xnode "Read/Write Control"("FPGA VI Reference In"=w640, "error in"=w639, "PWM Duty Cycle (Ticks) 51"=w637) -> ("FPGA VI Reference Out"=w642:refnum<k20>, "error out"=w641:errorcluster, "9401/Slot 3 Error Code"=w643:i32)
                    "/D51" <- w635
                  }
                  frame 52 {
                    n551 = Multiply(x=w644, y=w645) -> (x*y=w647:dbl)
                    n552 = To Long Integer(number=w647) -> (32bit integer=w646:i32)
                    n553 = xnode "Read/Write Control"("FPGA VI Reference In"=w649, "error in"=w648, "PWM Duty Cycle (Ticks) 52"=w646) -> ("FPGA VI Reference Out"=w651:refnum<k20>, "error out"=w650:errorcluster, "9401/Slot 3 Error Code"=w652:i32)
                    "/D52" <- w644
                  }
                  frame 53 {
                    n554 = Multiply(x=w653, y=w654) -> (x*y=w656:dbl)
                    n555 = To Long Integer(number=w656) -> (32bit integer=w655:i32)
                    n556 = xnode "Read/Write Control"("FPGA VI Reference In"=w658, "error in"=w657, "PWM Duty Cycle (Ticks) 53"=w655) -> ("FPGA VI Reference Out"=w660:refnum<k20>, "error out"=w659:errorcluster, "9401/Slot 3 Error Code"=w661:i32)
                    "/D53" <- w653
                  }
                  frame 54 {
                    n557 = Multiply(x=w662, y=w663) -> (x*y=w665:dbl)
                    n558 = To Long Integer(number=w665) -> (32bit integer=w664:i32)
                    n559 = xnode "Read/Write Control"("FPGA VI Reference In"=w667, "error in"=w666, "PWM Duty Cycle (Ticks) 54"=w664) -> ("FPGA VI Reference Out"=w669:refnum<k20>, "error out"=w668:errorcluster, "9401/Slot 3 Error Code"=w670:i32)
                    "/D54" <- w662
                  }
                  frame 55 {
                    n560 = Multiply(x=w671, y=w672) -> (x*y=w674:dbl)
                    n561 = To Long Integer(number=w674) -> (32bit integer=w673:i32)
                    n562 = xnode "Read/Write Control"("FPGA VI Reference In"=w676, "error in"=w675, "PWM Duty Cycle (Ticks) 55"=w673) -> ("FPGA VI Reference Out"=w678:refnum<k20>, "error out"=w677:errorcluster, "9401/Slot 3 Error Code"=w679:i32)
                    "/D55" <- w671
                  }
                  frame 56 {
                    n563 = Multiply(x=w680, y=w681) -> (x*y=w683:dbl)
                    n564 = To Long Integer(number=w683) -> (32bit integer=w682:i32)
                    n565 = xnode "Read/Write Control"("FPGA VI Reference In"=w685, "error in"=w684, "PWM Duty Cycle (Ticks) 56"=w682) -> ("FPGA VI Reference Out"=w687:refnum<k20>, "error out"=w686:errorcluster, "9401/Slot 3 Error Code"=w688:i32)
                    "/D56" <- w680
                  }
                  frame 57 {
                    n566 = Multiply(x=w689, y=w690) -> (x*y=w692:dbl)
                    n567 = To Long Integer(number=w692) -> (32bit integer=w691:i32)
                    n568 = xnode "Read/Write Control"("FPGA VI Reference In"=w694, "error in"=w693, "PWM Duty Cycle (Ticks) 57"=w691) -> ("FPGA VI Reference Out"=w696:refnum<k20>, "error out"=w695:errorcluster, "9401/Slot 3 Error Code"=w697:i32)
                    "/D57" <- w689
                  }
                  frame 58 {
                    n569 = Multiply(x=w698, y=w699) -> (x*y=w701:dbl)
                    n570 = To Long Integer(number=w701) -> (32bit integer=w700:i32)
                    n571 = xnode "Read/Write Control"("FPGA VI Reference In"=w703, "error in"=w702, "PWM Duty Cycle (Ticks) 58"=w700) -> ("FPGA VI Reference Out"=w705:refnum<k20>, "error out"=w704:errorcluster, "9401/Slot 3 Error Code"=w706:i32)
                    "/D58" <- w698
                  }
                  frame 59 {
                    n572 = Not Equal To 0?(x=w707) -> (x != 0?=w708:bool)
                    n573 = case shown="True" w708 {
                      tunnel: w707 -> [w719 _]
                      tunnel: [w727 w730] -> w714
                      tunnel: [w726 w729] -> w713
                      tunnel: [w725 0 ("9401/Slot 3 Error Code")] -> w712
                      tunnel: w711 -> [w724 w730]
                      tunnel: w710 -> [w723 w729]
                      tunnel: w709 -> [w715 _]
                      frame True {
                        n574 = Divide(x=w719, y=20.0) -> (x/y=w721:dbl)
                        n575 = Add(x=w721, y=0.05) -> (x+y=w716:dbl)
                        n576 = Multiply(x=w715, y=w716) -> (x*y=w717:dbl)
                        n577 = To Long Integer(number=w717) -> (32bit integer=w718:i32)
                        n578 = xnode "Read/Write Control"("FPGA VI Reference In"=w724, "error in"=w723, "PWM Duty Cycle (Ticks) 59"=w718) -> ("FPGA VI Reference Out"=w727:refnum<k20>, "error out"=w726:errorcluster, "9401/Slot 3 Error Code"=w725:i32)
                        "/D59" <- w719
                      }
                      frame False {
                      }
                    }
                  }
                  frame 60 {
                    n579 = Not Equal To 0?(x=w731) -> (x != 0?=w732:bool)
                    n580 = case shown="True" w732 {
                      tunnel: w731 -> [w743 _]
                      tunnel: [w751 w754] -> w738
                      tunnel: [w750 w753] -> w737
                      tunnel: [w749 0 ("9401/Slot 3 Error Code")] -> w736
                      tunnel: w735 -> [w748 w754]
                      tunnel: w734 -> [w747 w753]
                      tunnel: w733 -> [w739 _]
                      frame True {
                        n581 = Divide(x=w743, y=20.0) -> (x/y=w745:dbl)
                        n582 = Add(x=w745, y=0.05) -> (x+y=w740:dbl)
                        n583 = Multiply(x=w739, y=w740) -> (x*y=w741:dbl)
                        n584 = To Long Integer(number=w741) -> (32bit integer=w742:i32)
                        n585 = xnode "Read/Write Control"("FPGA VI Reference In"=w748, "error in"=w747, "PWM Duty Cycle (Ticks) 60"=w742) -> ("FPGA VI Reference Out"=w751:refnum<k20>, "error out"=w750:errorcluster, "9401/Slot 3 Error Code"=w749:i32)
                        "/D60" <- w743
                      }
                      frame False {
                      }
                    }
                  }
                  frame 61 {
                    n586 = Not Equal To 0?(x=w755) -> (x != 0?=w756:bool)
                    n587 = case shown="True" w756 {
                      tunnel: w755 -> [w767 _]
                      tunnel: [w775 w778] -> w762
                      tunnel: [w774 w777] -> w761
                      tunnel: [w773 0 ("9401/Slot 3 Error Code")] -> w760
                      tunnel: w759 -> [w772 w778]
                      tunnel: w758 -> [w771 w777]
                      tunnel: w757 -> [w763 _]
                      frame True {
                        n588 = Divide(x=w767, y=20.0) -> (x/y=w769:dbl)
                        n589 = Add(x=w769, y=0.05) -> (x+y=w764:dbl)
                        n590 = Multiply(x=w763, y=w764) -> (x*y=w765:dbl)
                        n591 = To Long Integer(number=w765) -> (32bit integer=w766:i32)
                        n592 = xnode "Read/Write Control"("FPGA VI Reference In"=w772, "error in"=w771, "PWM Duty Cycle (Ticks) 61"=w766) -> ("FPGA VI Reference Out"=w775:refnum<k20>, "error out"=w774:errorcluster, "9401/Slot 3 Error Code"=w773:i32)
                        "/D61" <- w767
                      }
                      frame False {
                      }
                    }
                  }
                  frame 62 {
                    n593 = Not Equal To 0?(x=w779) -> (x != 0?=w780:bool)
                    n594 = case shown="True" w780 {
                      tunnel: w779 -> [w791 _]
                      tunnel: [w799 w802] -> w786
                      tunnel: [w798 w801] -> w785
                      tunnel: [w797 0 ("9401/Slot 3 Error Code")] -> w784
                      tunnel: w781 -> [w796 w802]
                      tunnel: w782 -> [w795 w801]
                      tunnel: w783 -> [w787 _]
                      frame True {
                        n595 = Divide(x=w791, y=20.0) -> (x/y=w793:dbl)
                        n596 = Add(x=w793, y=0.05) -> (x+y=w788:dbl)
                        n597 = Multiply(x=w787, y=w788) -> (x*y=w789:dbl)
                        n598 = To Long Integer(number=w789) -> (32bit integer=w790:i32)
                        n599 = xnode "Read/Write Control"("FPGA VI Reference In"=w796, "error in"=w795, "PWM Duty Cycle (Ticks) 62"=w790) -> ("FPGA VI Reference Out"=w799:refnum<k20>, "error out"=w798:errorcluster, "9401/Slot 3 Error Code"=w797:i32)
                        "/D62" <- w791
                      }
                      frame False {
                      }
                    }
                  }
                  frame 63 {
                    n600 = Not Equal To 0?(x=w803) -> (x != 0?=w804:bool)
                    n601 = case shown="True" w804 {
                      tunnel: w803 -> [w815 _]
                      tunnel: [w823 w826] -> w810
                      tunnel: [w822 w825] -> w809
                      tunnel: [w821 0 ("9401/Slot 3 Error Code")] -> w808
                      tunnel: w805 -> [w820 w826]
                      tunnel: w806 -> [w819 w825]
                      tunnel: w807 -> [w811 _]
                      frame True {
                        n602 = Divide(x=w815, y=20.0) -> (x/y=w817:dbl)
                        n603 = Add(x=w817, y=0.05) -> (x+y=w812:dbl)
                        n604 = Multiply(x=w811, y=w812) -> (x*y=w813:dbl)
                        n605 = To Long Integer(number=w813) -> (32bit integer=w814:i32)
                        n606 = xnode "Read/Write Control"("FPGA VI Reference In"=w820, "error in"=w819, "PWM Duty Cycle (Ticks) 63"=w814) -> ("FPGA VI Reference Out"=w823:refnum<k20>, "error out"=w822:errorcluster, "9401/Slot 3 Error Code"=w821:i32)
                        "/D63" <- w815
                      }
                      frame False {
                      }
                    }
                  }
                  frame 64 {
                    n607 = Not Equal To 0?(x=w827) -> (x != 0?=w828:bool)
                    n608 = case shown="True" w828 {
                      tunnel: w827 -> [w839 _]
                      tunnel: [w847 w850] -> w834
                      tunnel: [w846 w849] -> w833
                      tunnel: [w845 0 ("9401/Slot 3 Error Code")] -> w832
                      tunnel: w831 -> [w844 w850]
                      tunnel: w830 -> [w843 w849]
                      tunnel: w829 -> [w835 _]
                      frame True {
                        n609 = Divide(x=w839, y=20.0) -> (x/y=w841:dbl)
                        n610 = Add(x=w841, y=0.05) -> (x+y=w836:dbl)
                        n611 = Multiply(x=w835, y=w836) -> (x*y=w837:dbl)
                        n612 = To Long Integer(number=w837) -> (32bit integer=w838:i32)
                        n613 = xnode "Read/Write Control"("FPGA VI Reference In"=w844, "error in"=w843, "PWM Duty Cycle (Ticks) 64"=w838) -> ("FPGA VI Reference Out"=w847:refnum<k20>, "error out"=w846:errorcluster, "9401/Slot 3 Error Code"=w845:i32)
                        "/D64" <- w839
                      }
                      frame False {
                      }
                    }
                  }
                  frame 65 {
                    n614 = for {
                      N: 59 -> [_]
                      shift-right: [w862] -> w855
                      shift-left: w853 -> [w859]
                      shift-right: [w861] -> w854
                      shift-left: _ -> [_]
                      shift-right: [w863] -> w856
                      shift-left: w852 -> [w860]
                      i -> [w858]
                      n615 = case shown="0, Default" w858 {
                        tunnel: w860 -> [w866 w872 w875 w880 w890 w896 w902 w908 w911 w917 w926 w932 w938 w944 w950 w956 w962 w968 w974 w980 w986 w992 w998 w1004 w1010 w1016 w1022 w1028 w1034 w1040 w1046 w1052 w1058 w1064 w1070 w1076 w1078 w1088 w1094 w1100 w1106 w1112 w1118 w1124 w1130 w1136 w1142 w1148 w1154 w1160 w1166 w1172 w1178 w1184 w1190 w1196 w1202 w1208 w1214]
                        tunnel: [0 ("9401/Slot 3 Error Code") w871 w876 w881 w886 w892 w898 w906 w912 w918 w922 w928 w934 w940 w946 w952 w958 w964 w971 w976 w982 w988 w994 w1000 w1006 w1012 w1018 w1024 w1030 w1036 w1042 w1048 w1054 w1060 w1066 w1072 w1079 w1084 w1090 w1096 w1102 w1108 w1114 w1120 w1126 w1132 w1138 w1144 w1150 w1156 w1162 w1168 w1174 w1180 w1186 w1192 w1198 w1204 w1210] -> w861
                        tunnel: [w866 w869 w878 w883 w888 w894 w900 w904 w914 w920 w924 w930 w936 w942 w948 w954 w960 w966 w970 w978 w984 w990 w996 w1002 w1008 w1014 w1020 w1026 w1032 w1038 w1044 w1050 w1056 w1062 w1068 w1074 w1081 w1086 w1092 w1098 w1104 w1110 w1116 w1122 w1128 w1134 w1140 w1146 w1152 w1158 w1164 w1170 w1176 w1182 w1188 w1194 w1200 w1206 w1212] -> w863
                        tunnel: w859 -> [w864 w870 w874 w884 w889 w895 w901 w907 w910 w916 w925 w931 w937 w943 w949 w955 w961 w967 w973 w979 w985 w991 w997 w1003 w1009 w1015 w1021 w1027 w1033 w1039 w1045 w1051 w1057 w1063 w1069 w1075 w1082 w1087 w1093 w1099 w1105 w1111 w1117 w1123 w1129 w1135 w1141 w1147 w1153 w1159 w1165 w1171 w1177 w1183 w1189 w1195 w1201 w1207 w1213]
                        tunnel: [w864 w868 w877 w882 w887 w893 w899 w905 w913 w919 w923 w929 w935 w941 w947 w953 w959 w965 w972 w977 w983 w989 w995 w1001 w1007 w1013 w1019 w1025 w1031 w1037 w1043 w1049 w1055 w1061 w1067 w1073 w1080 w1085 w1091 w1097 w1103 w1109 w1115 w1121 w1127 w1133 w1139 w1145 w1151 w1157 w1163 w1169 w1175 w1181 w1187 w1193 w1199 w1205 w1211] -> w862
                        tunnel: 0 -> [_ w867 w873 w879 w885 w891 w897 w903 w909 w915 w921 w927 w933 w939 w945 w951 w957 w963 w969 w975 w981 w987 w993 w999 w1005 w1011 w1017 w1023 w1029 w1035 w1041 w1047 w1053 w1059 w1065 w1071 w1077 w1083 w1089 w1095 w1101 w1107 w1113 w1119 w1125 w1131 w1137 w1143 w1149 w1155 w1161 w1167 w1173 w1179 w1185 w1191 w1197 w1203 w1209]
                        frame 0, Default {
                        }
                        frame 1 {
                          n616 = xnode "Read/Write Control"("FPGA VI Reference In"=w872, "error in"=w870, "PWM Duty Cycle (Ticks) 1"=w867) -> ("FPGA VI Reference Out"=w869:refnum<k20>, "error out"=w868:errorcluster, "9401/Slot 3 Error Code"=w871:i32)
                          n617 = local write "/D1"(w867) -> ()
                        }
                        frame 2 {
                          n618 = xnode "Read/Write Control"("FPGA VI Reference In"=w875, "error in"=w874, "PWM Duty Cycle (Ticks) 2"=w873) -> ("FPGA VI Reference Out"=w878:refnum<k20>, "error out"=w877:errorcluster, "9401/Slot 3 Error Code"=w876:i32)
                          n619 = local write "/D2"(w873) -> ()
                        }
                        frame 3 {
                          n620 = xnode "Read/Write Control"("FPGA VI Reference In"=w880, "error in"=w884, "PWM Duty Cycle (Ticks) 3"=w879) -> ("FPGA VI Reference Out"=w883:refnum<k20>, "error out"=w882:errorcluster, "9401/Slot 3 Error Code"=w881:i32)
                          n621 = local write "/D3"(w879) -> ()
                        }
                        frame 4 {
                          n622 = xnode "Read/Write Control"("FPGA VI Reference In"=w890, "error in"=w889, "PWM Duty Cycle (Ticks) 4"=w885) -> ("FPGA VI Reference Out"=w888:refnum<k20>, "error out"=w887:errorcluster, "9401/Slot 3 Error Code"=w886:i32)
                          n623 = local write "/D4"(w885) -> ()
                        }
                        frame 5 {
                          n624 = xnode "Read/Write Control"("FPGA VI Reference In"=w896, "error in"=w895, "PWM Duty Cycle (Ticks) 5"=w891) -> ("FPGA VI Reference Out"=w894:refnum<k20>, "error out"=w893:errorcluster, "9401/Slot 3 Error Code"=w892:i32)
                          n625 = local write "/D5"(w891) -> ()
                        }
                        frame 6 {
                          n626 = xnode "Read/Write Control"("FPGA VI Reference In"=w902, "error in"=w901, "PWM Duty Cycle (Ticks) 6"=w897) -> ("FPGA VI Reference Out"=w900:refnum<k20>, "error out"=w899:errorcluster, "9401/Slot 3 Error Code"=w898:i32)
                          n627 = local write "/D6"(w897) -> ()
                        }
                        frame 7 {
                          n628 = xnode "Read/Write Control"("FPGA VI Reference In"=w908, "error in"=w907, "PWM Duty Cycle (Ticks) 7"=w903) -> ("FPGA VI Reference Out"=w904:refnum<k20>, "error out"=w905:errorcluster, "9401/Slot 3 Error Code"=w906:i32)
                          n629 = local write "/D7"(w903) -> ()
                        }
                        frame 8 {
                          n630 = xnode "Read/Write Control"("FPGA VI Reference In"=w911, "error in"=w910, "PWM Duty Cycle (Ticks) 8"=w909) -> ("FPGA VI Reference Out"=w914:refnum<k20>, "error out"=w913:errorcluster, "9401/Slot 3 Error Code"=w912:i32)
                          n631 = local write "/D8"(w909) -> ()
                        }
                        frame 9 {
                          n632 = xnode "Read/Write Control"("FPGA VI Reference In"=w917, "error in"=w916, "PWM Duty Cycle (Ticks) 9"=w915) -> ("FPGA VI Reference Out"=w920:refnum<k20>, "error out"=w919:errorcluster, "9401/Slot 3 Error Code"=w918:i32)
                          n633 = local write "/D9"(w915) -> ()
                        }
                        frame 10 {
                          n634 = xnode "Read/Write Control"("FPGA VI Reference In"=w926, "error in"=w925, "PWM Duty Cycle (Ticks) 10"=w921) -> ("FPGA VI Reference Out"=w924:refnum<k20>, "error out"=w923:errorcluster, "9401/Slot 3 Error Code"=w922:i32)
                          n635 = local write "/D10"(w921) -> ()
                        }
                        frame 11 {
                          n636 = xnode "Read/Write Control"("FPGA VI Reference In"=w932, "error in"=w931, "PWM Duty Cycle (Ticks) 11"=w927) -> ("FPGA VI Reference Out"=w930:refnum<k20>, "error out"=w929:errorcluster, "9401/Slot 3 Error Code"=w928:i32)
                          n637 = local write "/D11"(w927) -> ()
                        }
                        frame 12 {
                          n638 = xnode "Read/Write Control"("FPGA VI Reference In"=w938, "error in"=w937, "PWM Duty Cycle (Ticks) 12"=w933) -> ("FPGA VI Reference Out"=w936:refnum<k20>, "error out"=w935:errorcluster, "9401/Slot 3 Error Code"=w934:i32)
                          n639 = local write "/D12"(w933) -> ()
                        }
                        frame 13 {
                          n640 = xnode "Read/Write Control"("FPGA VI Reference In"=w944, "error in"=w943, "PWM Duty Cycle (Ticks) 13"=w939) -> ("FPGA VI Reference Out"=w942:refnum<k20>, "error out"=w941:errorcluster, "9401/Slot 3 Error Code"=w940:i32)
                          n641 = local write "/D13"(w939) -> ()
                        }
                        frame 14 {
                          n642 = xnode "Read/Write Control"("FPGA VI Reference In"=w950, "error in"=w949, "PWM Duty Cycle (Ticks) 14"=w945) -> ("FPGA VI Reference Out"=w948:refnum<k20>, "error out"=w947:errorcluster, "9401/Slot 3 Error Code"=w946:i32)
                          n643 = local write "/D14"(w945) -> ()
                        }
                        frame 15 {
                          n644 = xnode "Read/Write Control"("FPGA VI Reference In"=w956, "error in"=w955, "PWM Duty Cycle (Ticks) 15"=w951) -> ("FPGA VI Reference Out"=w954:refnum<k20>, "error out"=w953:errorcluster, "9401/Slot 3 Error Code"=w952:i32)
                          n645 = local write "/D15"(w951) -> ()
                        }
                        frame 16 {
                          n646 = xnode "Read/Write Control"("FPGA VI Reference In"=w962, "error in"=w961, "PWM Duty Cycle (Ticks) 16"=w957) -> ("FPGA VI Reference Out"=w960:refnum<k20>, "error out"=w959:errorcluster, "9401/Slot 3 Error Code"=w958:i32)
                          n647 = local write "/D16"(w957) -> ()
                        }
                        frame 17 {
                          n648 = xnode "Read/Write Control"("FPGA VI Reference In"=w968, "error in"=w967, "PWM Duty Cycle (Ticks) 17"=w963) -> ("FPGA VI Reference Out"=w966:refnum<k20>, "error out"=w965:errorcluster, "9401/Slot 3 Error Code"=w964:i32)
                          n649 = local write "/D17"(w963) -> ()
                        }
                        frame 18 {
                          n650 = xnode "Read/Write Control"("FPGA VI Reference In"=w974, "error in"=w973, "PWM Duty Cycle (Ticks) 18"=w969) -> ("FPGA VI Reference Out"=w970:refnum<k20>, "error out"=w972:errorcluster, "9401/Slot 3 Error Code"=w971:i32)
                          n651 = local write "/D18"(w969) -> ()
                        }
                        frame 19 {
                          n652 = xnode "Read/Write Control"("FPGA VI Reference In"=w980, "error in"=w979, "PWM Duty Cycle (Ticks) 19"=w975) -> ("FPGA VI Reference Out"=w978:refnum<k20>, "error out"=w977:errorcluster, "9401/Slot 3 Error Code"=w976:i32)
                          n653 = local write "/D19"(w975) -> ()
                        }
                        frame 20 {
                          n654 = xnode "Read/Write Control"("FPGA VI Reference In"=w986, "error in"=w985, "PWM Duty Cycle (Ticks) 20"=w981) -> ("FPGA VI Reference Out"=w984:refnum<k20>, "error out"=w983:errorcluster, "9401/Slot 3 Error Code"=w982:i32)
                          n655 = local write "/D20"(w981) -> ()
                        }
                        frame 21 {
                          n656 = xnode "Read/Write Control"("FPGA VI Reference In"=w992, "error in"=w991, "PWM Duty Cycle (Ticks) 21"=w987) -> ("FPGA VI Reference Out"=w990:refnum<k20>, "error out"=w989:errorcluster, "9401/Slot 3 Error Code"=w988:i32)
                          n657 = local write "/D21"(w987) -> ()
                        }
                        frame 22 {
                          n658 = xnode "Read/Write Control"("FPGA VI Reference In"=w998, "error in"=w997, "PWM Duty Cycle (Ticks) 22"=w993) -> ("FPGA VI Reference Out"=w996:refnum<k20>, "error out"=w995:errorcluster, "9401/Slot 3 Error Code"=w994:i32)
                          n659 = local write "/D22"(w993) -> ()
                        }
                        frame 23 {
                          n660 = xnode "Read/Write Control"("FPGA VI Reference In"=w1004, "error in"=w1003, "PWM Duty Cycle (Ticks) 23"=w999) -> ("FPGA VI Reference Out"=w1002:refnum<k20>, "error out"=w1001:errorcluster, "9401/Slot 3 Error Code"=w1000:i32)
                          n661 = local write "/D23"(w999) -> ()
                        }
                        frame 24 {
                          n662 = xnode "Read/Write Control"("FPGA VI Reference In"=w1010, "error in"=w1009, "PWM Duty Cycle (Ticks) 24"=w1005) -> ("FPGA VI Reference Out"=w1008:refnum<k20>, "error out"=w1007:errorcluster, "9401/Slot 3 Error Code"=w1006:i32)
                          n663 = local write "/D24"(w1005) -> ()
                        }
                        frame 25 {
                          n664 = local write "/D25"(w1011) -> ()
                          n665 = xnode "Read/Write Control"("FPGA VI Reference In"=w1016, "error in"=w1015, "PWM Duty Cycle (Ticks) 25"=w1011) -> ("FPGA VI Reference Out"=w1014:refnum<k20>, "error out"=w1013:errorcluster, "9401/Slot 3 Error Code"=w1012:i32)
                        }
                        frame 26 {
                          n666 = xnode "Read/Write Control"("FPGA VI Reference In"=w1022, "error in"=w1021, "PWM Duty Cycle (Ticks) 26"=w1017) -> ("FPGA VI Reference Out"=w1020:refnum<k20>, "error out"=w1019:errorcluster, "9401/Slot 3 Error Code"=w1018:i32)
                          n667 = local write "/D26"(w1017) -> ()
                        }
                        frame 27 {
                          n668 = xnode "Read/Write Control"("FPGA VI Reference In"=w1028, "error in"=w1027, "PWM Duty Cycle (Ticks) 27"=w1023) -> ("FPGA VI Reference Out"=w1026:refnum<k20>, "error out"=w1025:errorcluster, "9401/Slot 3 Error Code"=w1024:i32)
                          n669 = local write "/D27"(w1023) -> ()
                        }
                        frame 28 {
                          n670 = local write "/D28"(w1029) -> ()
                          n671 = xnode "Read/Write Control"("FPGA VI Reference In"=w1034, "error in"=w1033, "PWM Duty Cycle (Ticks) 28"=w1029) -> ("FPGA VI Reference Out"=w1032:refnum<k20>, "error out"=w1031:errorcluster, "9401/Slot 3 Error Code"=w1030:i32)
                        }
                        frame 29 {
                          n672 = xnode "Read/Write Control"("FPGA VI Reference In"=w1040, "error in"=w1039, "PWM Duty Cycle (Ticks) 29"=w1035) -> ("FPGA VI Reference Out"=w1038:refnum<k20>, "error out"=w1037:errorcluster, "9401/Slot 3 Error Code"=w1036:i32)
                          n673 = local write "/D29"(w1035) -> ()
                        }
                        frame 30 {
                          n674 = local write "/D30"(w1041) -> ()
                          n675 = xnode "Read/Write Control"("FPGA VI Reference In"=w1046, "error in"=w1045, "PWM Duty Cycle (Ticks) 30"=w1041) -> ("FPGA VI Reference Out"=w1044:refnum<k20>, "error out"=w1043:errorcluster, "9401/Slot 3 Error Code"=w1042:i32)
                        }
                        frame 31 {
                          n676 = local write "/D31"(w1047) -> ()
                          n677 = xnode "Read/Write Control"("FPGA VI Reference In"=w1052, "error in"=w1051, "PWM Duty Cycle (Ticks) 31"=w1047) -> ("FPGA VI Reference Out"=w1050:refnum<k20>, "error out"=w1049:errorcluster, "9401/Slot 3 Error Code"=w1048:i32)
                        }
                        frame 32 {
                          n678 = xnode "Read/Write Control"("FPGA VI Reference In"=w1058, "error in"=w1057, "PWM Duty Cycle (Ticks) 32"=w1053) -> ("FPGA VI Reference Out"=w1056:refnum<k20>, "error out"=w1055:errorcluster, "9401/Slot 3 Error Code"=w1054:i32)
                          n679 = local write "/D32"(w1053) -> ()
                        }
                        frame 33 {
                          n680 = local write "/D33"(w1059) -> ()
                          n681 = xnode "Read/Write Control"("FPGA VI Reference In"=w1064, "error in"=w1063, "PWM Duty Cycle (Ticks) 33"=w1059) -> ("FPGA VI Reference Out"=w1062:refnum<k20>, "error out"=w1061:errorcluster, "9401/Slot 3 Error Code"=w1060:i32)
                        }
                        frame 34 {
                          n682 = local write "/D34"(w1065) -> ()
                          n683 = xnode "Read/Write Control"("FPGA VI Reference In"=w1070, "error in"=w1069, "PWM Duty Cycle (Ticks) 34"=w1065) -> ("FPGA VI Reference Out"=w1068:refnum<k20>, "error out"=w1067:errorcluster, "9401/Slot 3 Error Code"=w1066:i32)
                        }
                        frame 35 {
                          n684 = local write "/D35"(w1071) -> ()
                          n685 = xnode "Read/Write Control"("FPGA VI Reference In"=w1076, "error in"=w1075, "PWM Duty Cycle (Ticks) 35"=w1071) -> ("FPGA VI Reference Out"=w1074:refnum<k20>, "error out"=w1073:errorcluster, "9401/Slot 3 Error Code"=w1072:i32)
                        }
                        frame 36 {
                          n686 = xnode "Read/Write Control"("FPGA VI Reference In"=w1078, "error in"=w1082, "PWM Duty Cycle (Ticks) 36"=w1077) -> ("FPGA VI Reference Out"=w1081:refnum<k20>, "error out"=w1080:errorcluster, "9401/Slot 3 Error Code"=w1079:i32)
                          n687 = local write "/D36"(w1077) -> ()
                        }
                        frame 37 {
                          n688 = xnode "Read/Write Control"("FPGA VI Reference In"=w1088, "error in"=w1087, "PWM Duty Cycle (Ticks) 37"=w1083) -> ("FPGA VI Reference Out"=w1086:refnum<k20>, "error out"=w1085:errorcluster, "9401/Slot 3 Error Code"=w1084:i32)
                          n689 = local write "/D37"(w1083) -> ()
                        }
                        frame 38 {
                          n690 = xnode "Read/Write Control"("FPGA VI Reference In"=w1094, "error in"=w1093, "PWM Duty Cycle (Ticks) 38"=w1089) -> ("FPGA VI Reference Out"=w1092:refnum<k20>, "error out"=w1091:errorcluster, "9401/Slot 3 Error Code"=w1090:i32)
                          n691 = local write "/D38"(w1089) -> ()
                        }
                        frame 39 {
                          n692 = xnode "Read/Write Control"("FPGA VI Reference In"=w1100, "error in"=w1099, "PWM Duty Cycle (Ticks) 39"=w1095) -> ("FPGA VI Reference Out"=w1098:refnum<k20>, "error out"=w1097:errorcluster, "9401/Slot 3 Error Code"=w1096:i32)
                          n693 = local write "/D39"(w1095) -> ()
                        }
                        frame 40 {
                          n694 = xnode "Read/Write Control"("FPGA VI Reference In"=w1106, "error in"=w1105, "PWM Duty Cycle (Ticks) 40"=w1101) -> ("FPGA VI Reference Out"=w1104:refnum<k20>, "error out"=w1103:errorcluster, "9401/Slot 3 Error Code"=w1102:i32)
                          n695 = local write "/D40"(w1101) -> ()
                        }
                        frame 41 {
                          n696 = xnode "Read/Write Control"("FPGA VI Reference In"=w1112, "error in"=w1111, "PWM Duty Cycle (Ticks) 41"=w1107) -> ("FPGA VI Reference Out"=w1110:refnum<k20>, "error out"=w1109:errorcluster, "9401/Slot 3 Error Code"=w1108:i32)
                          n697 = local write "/D41"(w1107) -> ()
                        }
                        frame 42 {
                          n698 = xnode "Read/Write Control"("FPGA VI Reference In"=w1118, "error in"=w1117, "PWM Duty Cycle (Ticks) 42"=w1113) -> ("FPGA VI Reference Out"=w1116:refnum<k20>, "error out"=w1115:errorcluster, "9401/Slot 3 Error Code"=w1114:i32)
                          n699 = local write "/D42"(w1113) -> ()
                        }
                        frame 43 {
                          n700 = xnode "Read/Write Control"("FPGA VI Reference In"=w1124, "error in"=w1123, "PWM Duty Cycle (Ticks) 43"=w1119) -> ("FPGA VI Reference Out"=w1122:refnum<k20>, "error out"=w1121:errorcluster, "9401/Slot 3 Error Code"=w1120:i32)
                          n701 = local write "/D43"(w1119) -> ()
                        }
                        frame 44 {
                          n702 = local write "/D44"(w1125) -> ()
                          n703 = xnode "Read/Write Control"("FPGA VI Reference In"=w1130, "error in"=w1129, "PWM Duty Cycle (Ticks) 44"=w1125) -> ("FPGA VI Reference Out"=w1128:refnum<k20>, "error out"=w1127:errorcluster, "9401/Slot 3 Error Code"=w1126:i32)
                        }
                        frame 45 {
                          n704 = local write "/D45"(w1131) -> ()
                          n705 = xnode "Read/Write Control"("FPGA VI Reference In"=w1136, "error in"=w1135, "PWM Duty Cycle (Ticks) 45"=w1131) -> ("FPGA VI Reference Out"=w1134:refnum<k20>, "error out"=w1133:errorcluster, "9401/Slot 3 Error Code"=w1132:i32)
                        }
                        frame 46 {
                          n706 = xnode "Read/Write Control"("FPGA VI Reference In"=w1142, "error in"=w1141, "PWM Duty Cycle (Ticks) 46"=w1137) -> ("FPGA VI Reference Out"=w1140:refnum<k20>, "error out"=w1139:errorcluster, "9401/Slot 3 Error Code"=w1138:i32)
                          n707 = local write "/D46"(w1137) -> ()
                        }
                        frame 47 {
                          n708 = xnode "Read/Write Control"("FPGA VI Reference In"=w1148, "error in"=w1147, "PWM Duty Cycle (Ticks) 47"=w1143) -> ("FPGA VI Reference Out"=w1146:refnum<k20>, "error out"=w1145:errorcluster, "9401/Slot 3 Error Code"=w1144:i32)
                          n709 = local write "/D47"(w1143) -> ()
                        }
                        frame 48 {
                          n710 = xnode "Read/Write Control"("FPGA VI Reference In"=w1154, "error in"=w1153, "PWM Duty Cycle (Ticks) 48"=w1149) -> ("FPGA VI Reference Out"=w1152:refnum<k20>, "error out"=w1151:errorcluster, "9401/Slot 3 Error Code"=w1150:i32)
                          n711 = local write "/D48"(w1149) -> ()
                        }
                        frame 49 {
                          n712 = local write "/D49"(w1155) -> ()
                          n713 = xnode "Read/Write Control"("FPGA VI Reference In"=w1160, "error in"=w1159, "PWM Duty Cycle (Ticks) 49"=w1155) -> ("FPGA VI Reference Out"=w1158:refnum<k20>, "error out"=w1157:errorcluster, "9401/Slot 3 Error Code"=w1156:i32)
                        }
                        frame 50 {
                          n714 = xnode "Read/Write Control"("FPGA VI Reference In"=w1166, "error in"=w1165, "PWM Duty Cycle (Ticks) 50"=w1161) -> ("FPGA VI Reference Out"=w1164:refnum<k20>, "error out"=w1163:errorcluster, "9401/Slot 3 Error Code"=w1162:i32)
                          n715 = local write "/D50"(w1161) -> ()
                        }
                        frame 51 {
                          n716 = xnode "Read/Write Control"("FPGA VI Reference In"=w1172, "error in"=w1171, "PWM Duty Cycle (Ticks) 51"=w1167) -> ("FPGA VI Reference Out"=w1170:refnum<k20>, "error out"=w1169:errorcluster, "9401/Slot 3 Error Code"=w1168:i32)
                          n717 = local write "/D51"(w1167) -> ()
                        }
                        frame 52 {
                          n718 = xnode "Read/Write Control"("FPGA VI Reference In"=w1178, "error in"=w1177, "PWM Duty Cycle (Ticks) 52"=w1173) -> ("FPGA VI Reference Out"=w1176:refnum<k20>, "error out"=w1175:errorcluster, "9401/Slot 3 Error Code"=w1174:i32)
                          n719 = local write "/D52"(w1173) -> ()
                        }
                        frame 53 {
                          n720 = xnode "Read/Write Control"("FPGA VI Reference In"=w1184, "error in"=w1183, "PWM Duty Cycle (Ticks) 53"=w1179) -> ("FPGA VI Reference Out"=w1182:refnum<k20>, "error out"=w1181:errorcluster, "9401/Slot 3 Error Code"=w1180:i32)
                          n721 = local write "/D53"(w1179) -> ()
                        }
                        frame 54 {
                          n722 = xnode "Read/Write Control"("FPGA VI Reference In"=w1190, "error in"=w1189, "PWM Duty Cycle (Ticks) 54"=w1185) -> ("FPGA VI Reference Out"=w1188:refnum<k20>, "error out"=w1187:errorcluster, "9401/Slot 3 Error Code"=w1186:i32)
                          n723 = local write "/D54"(w1185) -> ()
                        }
                        frame 55 {
                          n724 = xnode "Read/Write Control"("FPGA VI Reference In"=w1196, "error in"=w1195, "PWM Duty Cycle (Ticks) 55"=w1191) -> ("FPGA VI Reference Out"=w1194:refnum<k20>, "error out"=w1193:errorcluster, "9401/Slot 3 Error Code"=w1192:i32)
                          n725 = local write "/D55"(w1191) -> ()
                        }
                        frame 56 {
                          n726 = xnode "Read/Write Control"("FPGA VI Reference In"=w1202, "error in"=w1201, "PWM Duty Cycle (Ticks) 56"=w1197) -> ("FPGA VI Reference Out"=w1200:refnum<k20>, "error out"=w1199:errorcluster, "9401/Slot 3 Error Code"=w1198:i32)
                          n727 = local write "/D56"(w1197) -> ()
                        }
                        frame 57 {
                          n728 = xnode "Read/Write Control"("FPGA VI Reference In"=w1208, "error in"=w1207, "PWM Duty Cycle (Ticks) 57"=w1203) -> ("FPGA VI Reference Out"=w1206:refnum<k20>, "error out"=w1205:errorcluster, "9401/Slot 3 Error Code"=w1204:i32)
                          n729 = local write "/D57"(w1203) -> ()
                        }
                        frame 58 {
                          n730 = xnode "Read/Write Control"("FPGA VI Reference In"=w1214, "error in"=w1213, "PWM Duty Cycle (Ticks) 58"=w1209) -> ("FPGA VI Reference Out"=w1212:refnum<k20>, "error out"=w1211:errorcluster, "9401/Slot 3 Error Code"=w1210:i32)
                          n731 = local write "/D58"(w1209) -> ()
                        }
                      }
                    }
                  }
                }
              }
            }
          }
        }
      }
      n732 = Greater?(x=w101, y=w113) -> (0:w114:bool)
      n733 = Wait Until Next ms Multiple(millisecond multiple=u32 50) -> ()  [unwired: 1 out]
    }
    n734 = Unbundle By Name(w80) -> ("status"=w81:bool)
    n735 = Unbundle By Name(w89) -> ("status"=w92:bool)
    n736 = Not Equal To 0?(x=w87) -> (x != 0?=w91:bool)
    n737 = Bundle By Name(cluster=w89, "status"=w91, "code"=w87, "source"="9401/Slot 3") -> (w86:errorcluster)
    n738 = Or(x=w92, y=w91) -> (x .or. y?=w82:bool)
    n739 = Or(x=w82, y=w81) -> (x .or. y?=w83:bool)
  }
  n740 = UDP Close(connection ID=w16, 8:w18) -> (error out=w17:errorcluster)  [unwired: 1 out]
  n741 = xnode "Read/Write Control"("FPGA VI Reference In"=w10, "error in"=w11, "stop"=w9) -> ("FPGA VI Reference Out"=w15:refnum<k20>, "error out"=w14:errorcluster)
  n742 = call <vilib>:"Simple Error Handler.vi"("error in (no error)"=w17) -> ()  [unwired: 4 in, 5 out]
  n743 = xnode "Close FPGA VI Reference"("FPGA VI Reference In"=w15, "error in"=w14) -> ("error out"=w13:errorcluster)
  n744 = Merge Errors(w13, w8) -> (→"error fpga":errorcluster)
